vi "TCC_31_05_16_LIBRA.vi"() -> ()   [LabVIEW 2010]
doc: "Use this template to build a standard state machine design pattern. Each state executes code and determines which state to transition to. Contrast this design pattern with the User Interface Event Handler pattern, in which code executes in response to user actions. Contrast this design pattern also with the Queued Message Handler pattern, in which each message handling code can queue zero or more new messages."
uses:
  TCC_01_02_15.ctl
  <vilib>/Instr/_visa.llb/VISA Configure Serial Port (Instr).vi
  <vilib>/Utility/file.llb/Write To Spreadsheet File (DBL).vi
  <vilib>/Analysis/NI_AALBase.lvlib
panel:
  out "Quantidade de Passos N-1":sgl
  in  "port":u16=20551
  out "Resulting string (W)":string
  in  "COM PIC":refnum<visa-resource-name>
  in  "Quit":bool
  in  "Inicia Controle":bool
  out "Diferença em %":dbl
  in  "Potência max Laser":dbl
  out "Meter Serial Number 8":string
  in  "Location of FieldMax2Lib.dll in 8":path=path "C:/Windows/System32/FieldMax2Lib.dll"
  out "Meter Serial Number 7":string
  in  "Location of FieldMax2Lib.dll in 7":path=path "C:/Windows/System32/FieldMax2Lib.dll"
  out "Meter Serial Number 6":string
  out "Mínima Pot":dbl=0.009
  out "Meter Serial Number 5":string
  in  "Location of FieldMax2Lib.dll in 5":path=path "C:/Windows/System32/FieldMax2Lib.dll"
  out "Meter Serial Number 4":string
  in  "Location of FieldMax2Lib.dll in 4":path=path "C:/Windows/System32/FieldMax2Lib.dll"
  out "Meter Serial Number 3":string
  out "Motor Sensor":bool
  out "Motor Disco":bool
  out "Shutter ON (Verde)/ OFF (Vermelho)":bool
  out "Measurement\n (W)":dbl format="%0.8f"
  out "Desv.Padrão":dbl format="%.8f"
  out "Quantidade de Passos":sgl
  in  "Medida (W)":dbl=0.027000000700354576 min=0.027000000700354576 max=0.27000001072883606 step=0.0005000000237487257 format="%0.8f"
  in  "Setpoint (W)":dbl=0.027000000700354576 min=0.027000000700354576 max=0.27000001072883606 step=0.0005000000237487257
  out "i":i32
  out "Medida N-1 (W)":dbl=0.027000000700354576 min=0.027000000700354576 max=0.27000001072883606 step=0.0005000000237487257 format="%0.8f"
  out "DeltaP":dbl
  out "Coeficiente novo":dbl
  out "Inicia\nAutomático":bool
  in  "Mensagem de erro renviada":string
  out "Máxima Pot":dbl=0.145
  in  "service name":string="localhost"
  out "FS/AS?":string
  out "connection P3D ID out":refnum<k5>
  out "Erro TCP 3DP":errorcluster
  in  "Location of FieldMax2Lib.dll in 6":path=path "C:/Windows/System32/FieldMax2Lib.dll"
  out "Erro comando PIC":errorcluster
  in  "Location of FieldMax2Lib.dll in 3":path=path "C:/Windows/System32/FieldMax2Lib.dll"
  out "Comandos para o PIC":string
  out "return count":u32
  out "data out":string
  out "bytes written":i32
  out "Loop  2":i32
  out "initialized array  2":sgl[](array[numeric]) format="%#_8g"
  out "Loop":i32
  out "initialized array":sgl[](array[numeric]) format="%#_8g"
  out "N_passos string":string
  # "- Entradas do programa:"
  # "-Indicadores:"
  # "- Informações do medidor:"
  # "- Variáveis auxiliares:"
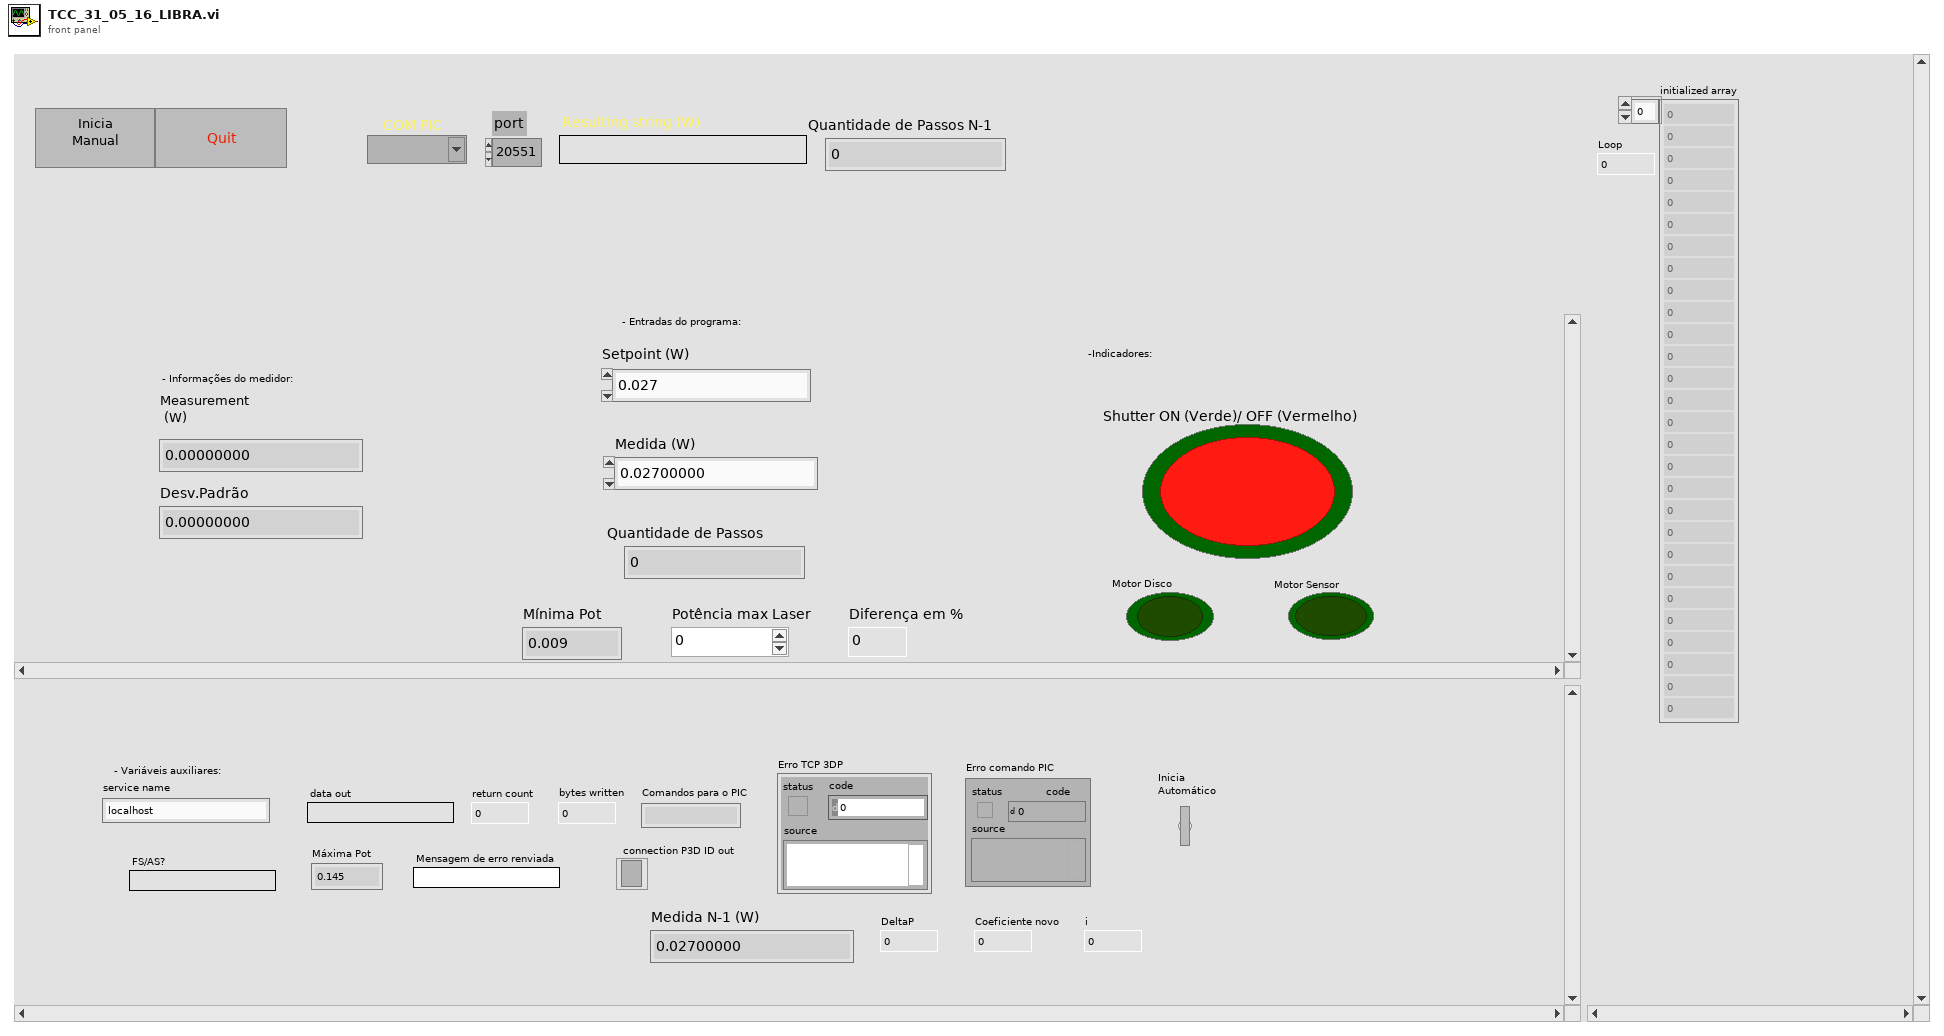
[diagram p1: front panel]
types:
  T1 = typedef "TCC_01_02_15.ctl" = enum16{"Receber Potencia", "Eventos", "Limites_P3D", "Limites_Manual", "Apenas Shutter", "Ajuste Manual", "Ajuste de Potência", "Stop"}
  T2 = enum8{"Enabled", "Disabled", "Disabled and Grayed Out"}
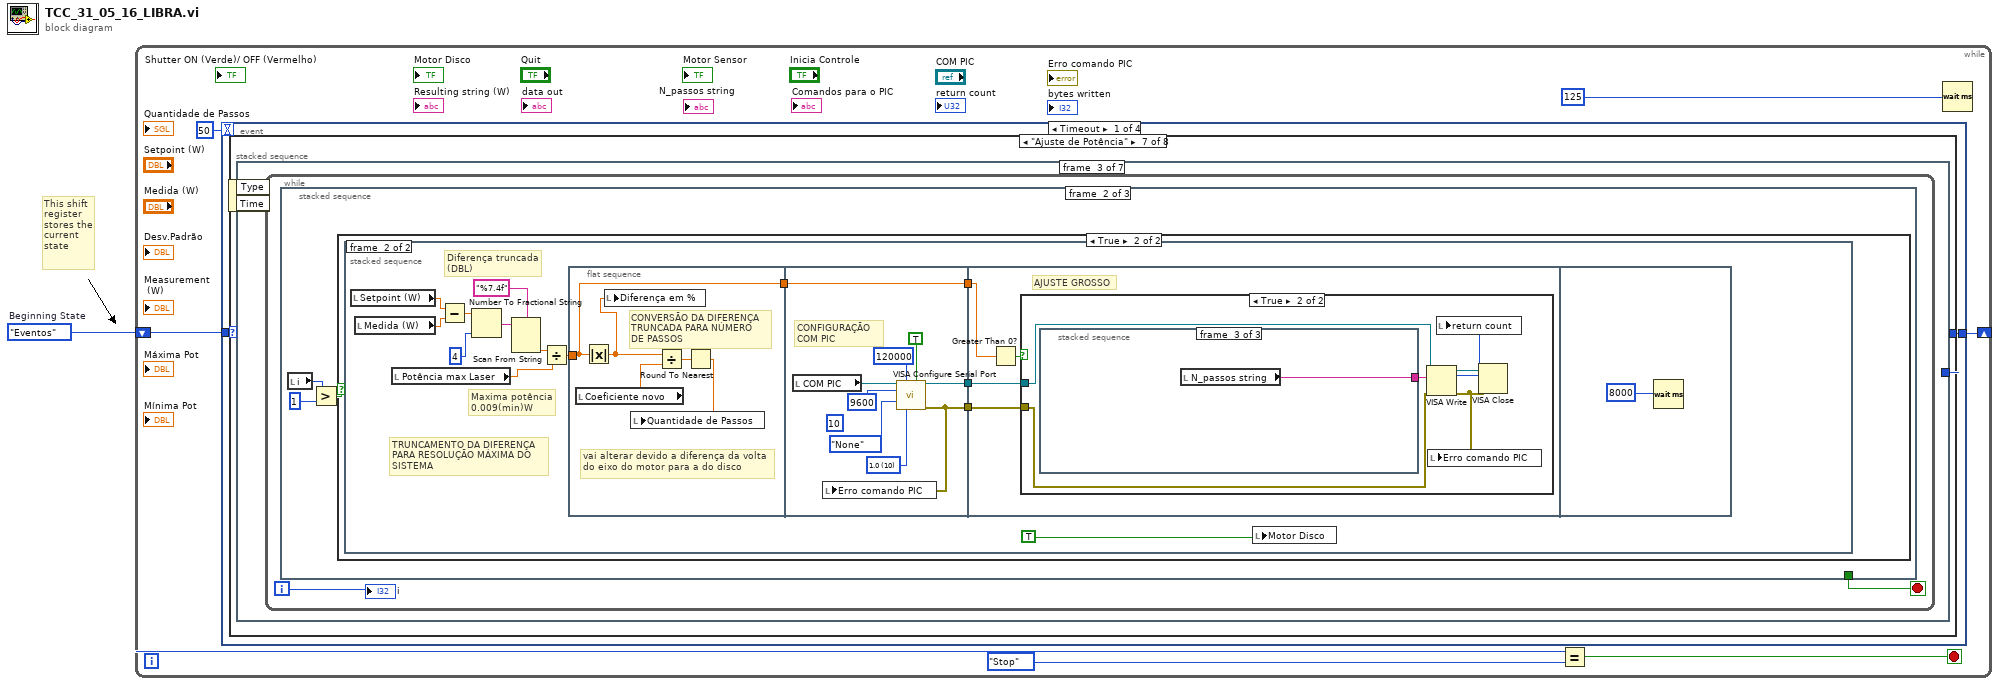
[diagram p0: block diagram]
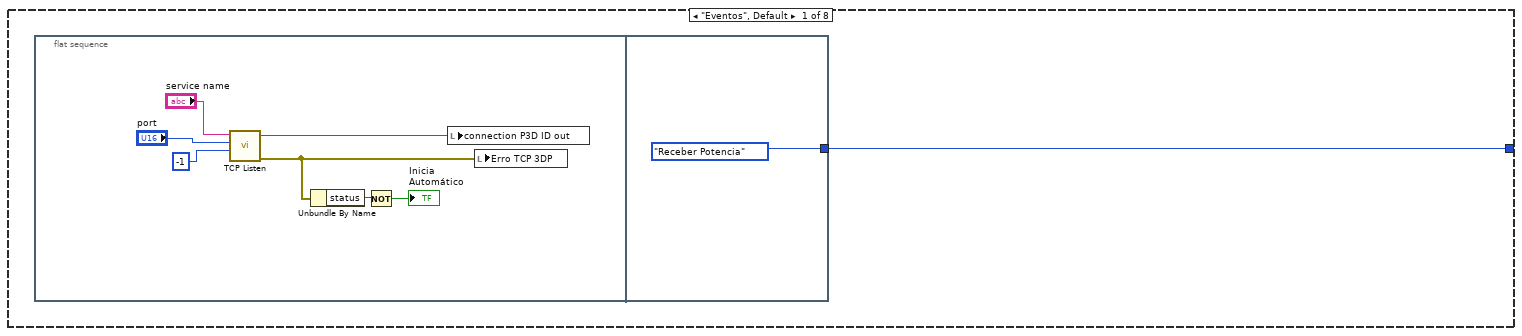
[diagram p2: hidden frame]
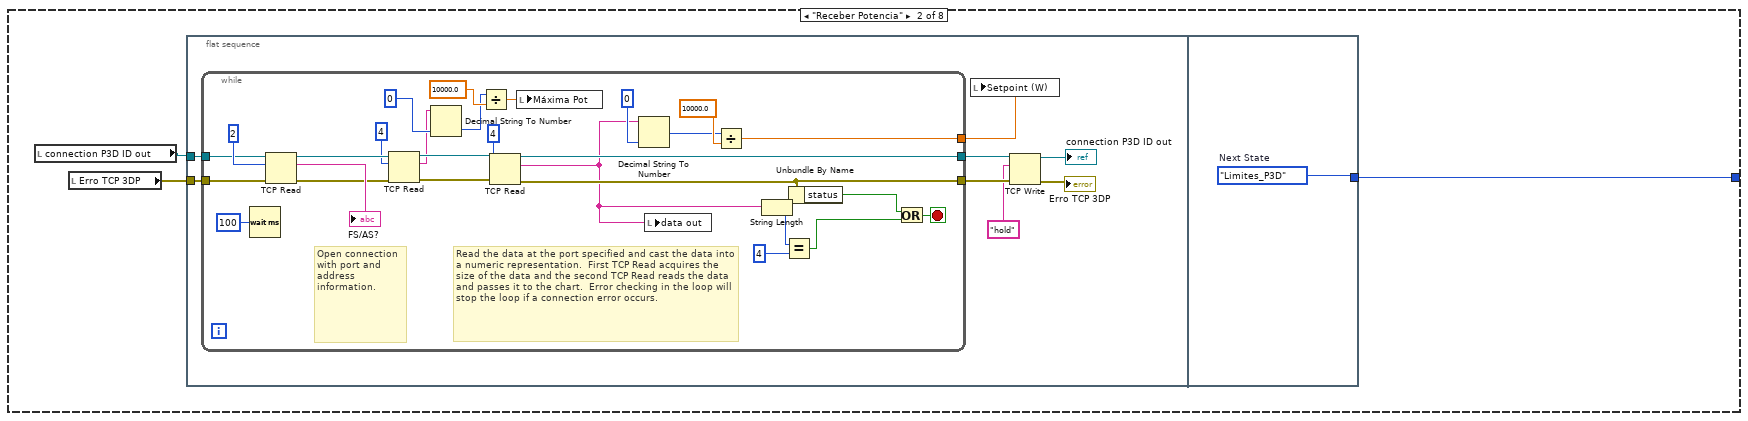
[diagram p3: hidden frame]
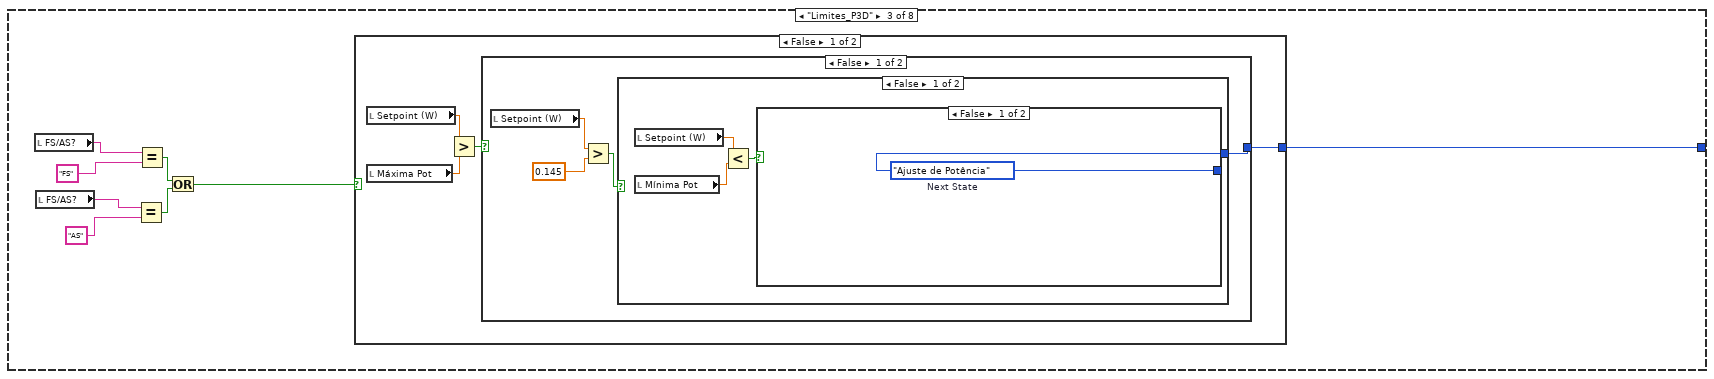
[diagram p4: hidden frame]
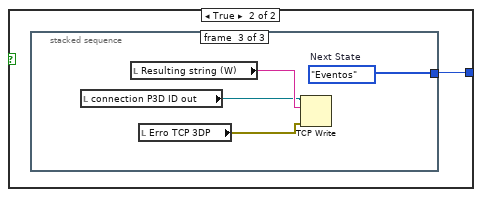
[diagram p5: hidden frame]
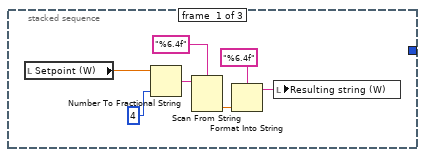
[diagram p6: hidden frame]
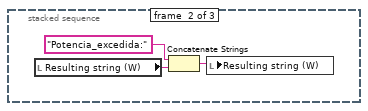
[diagram p7: hidden frame]
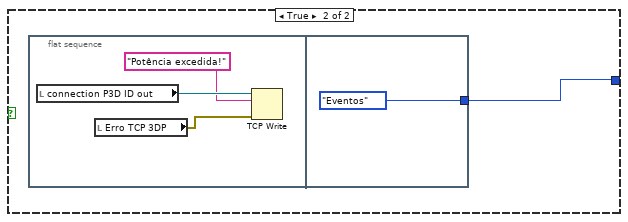
[diagram p8: hidden frame]
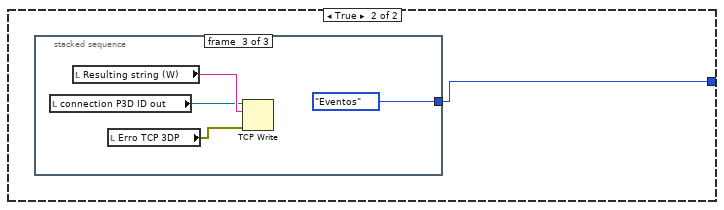
[diagram p9: hidden frame]
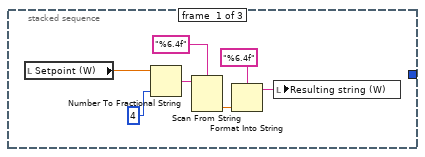
[diagram p10: hidden frame]
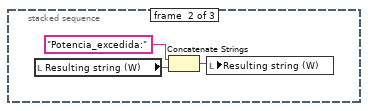
[diagram p11: hidden frame]
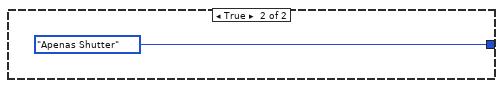
[diagram p12: hidden frame]
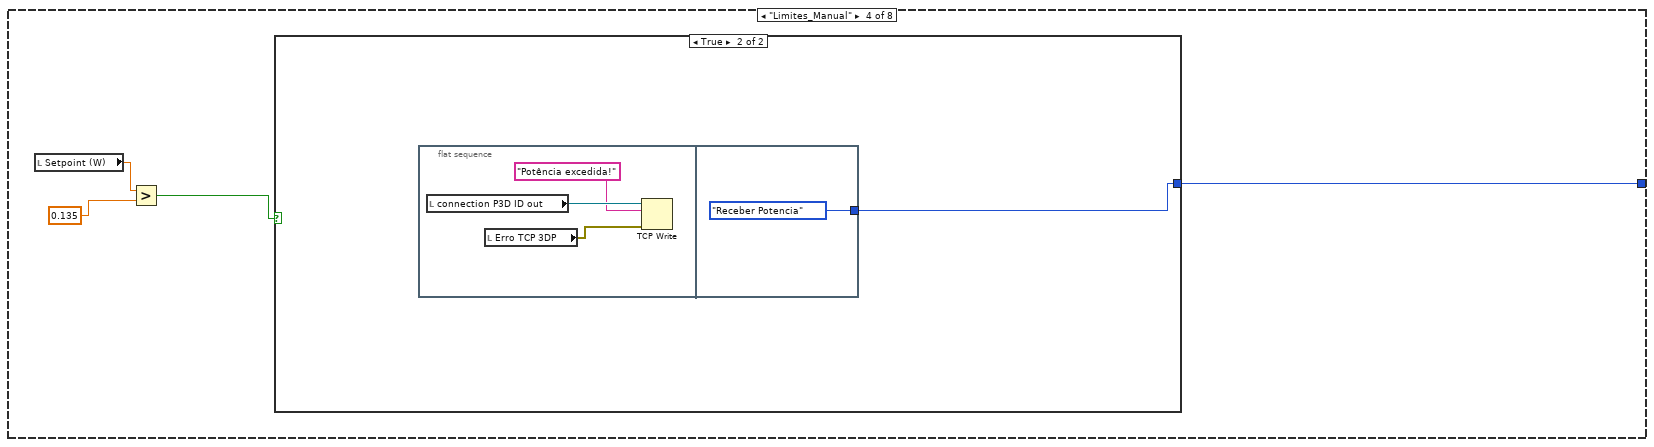
[diagram p13: hidden frame]
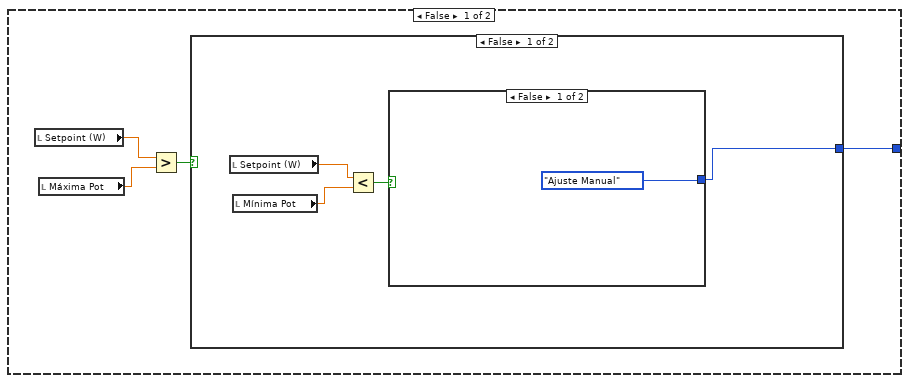
[diagram p14: hidden frame]
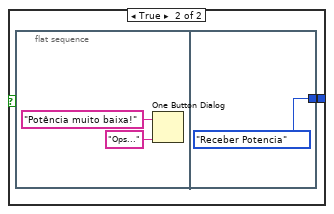
[diagram p15: hidden frame]
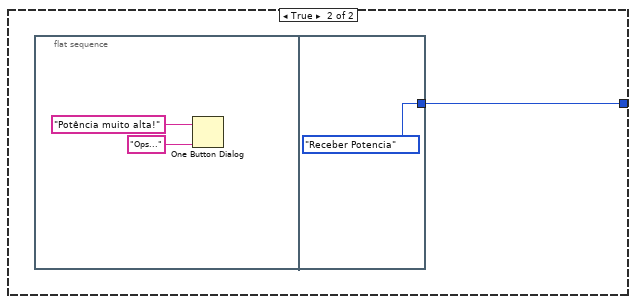
[diagram p16: hidden frame]
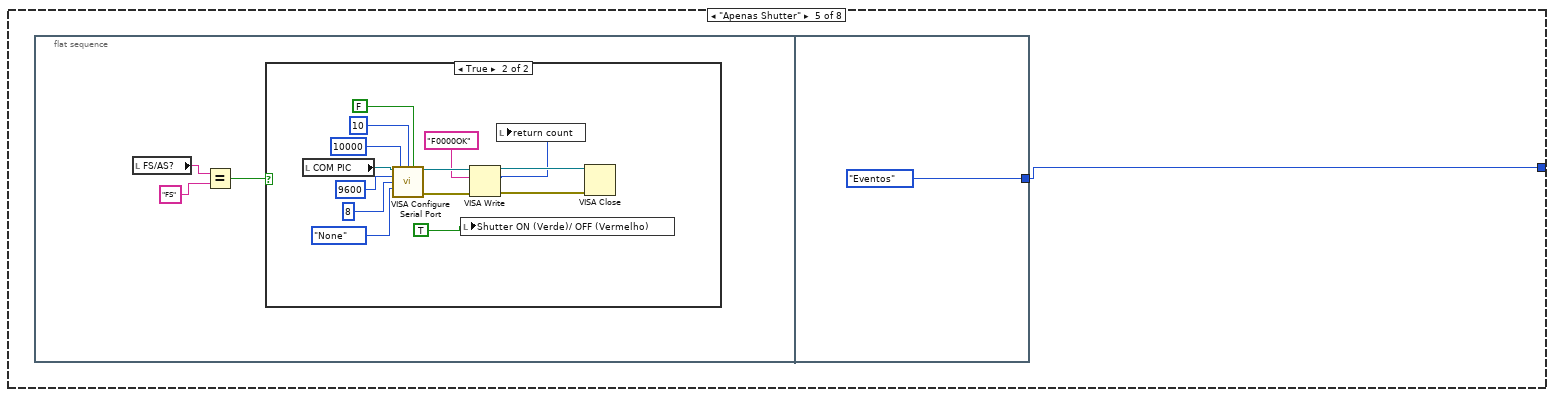
[diagram p17: hidden frame]
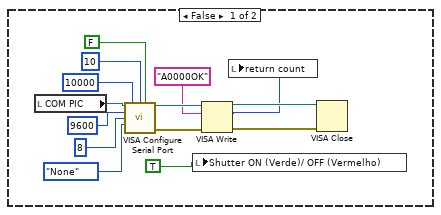
[diagram p18: hidden frame]
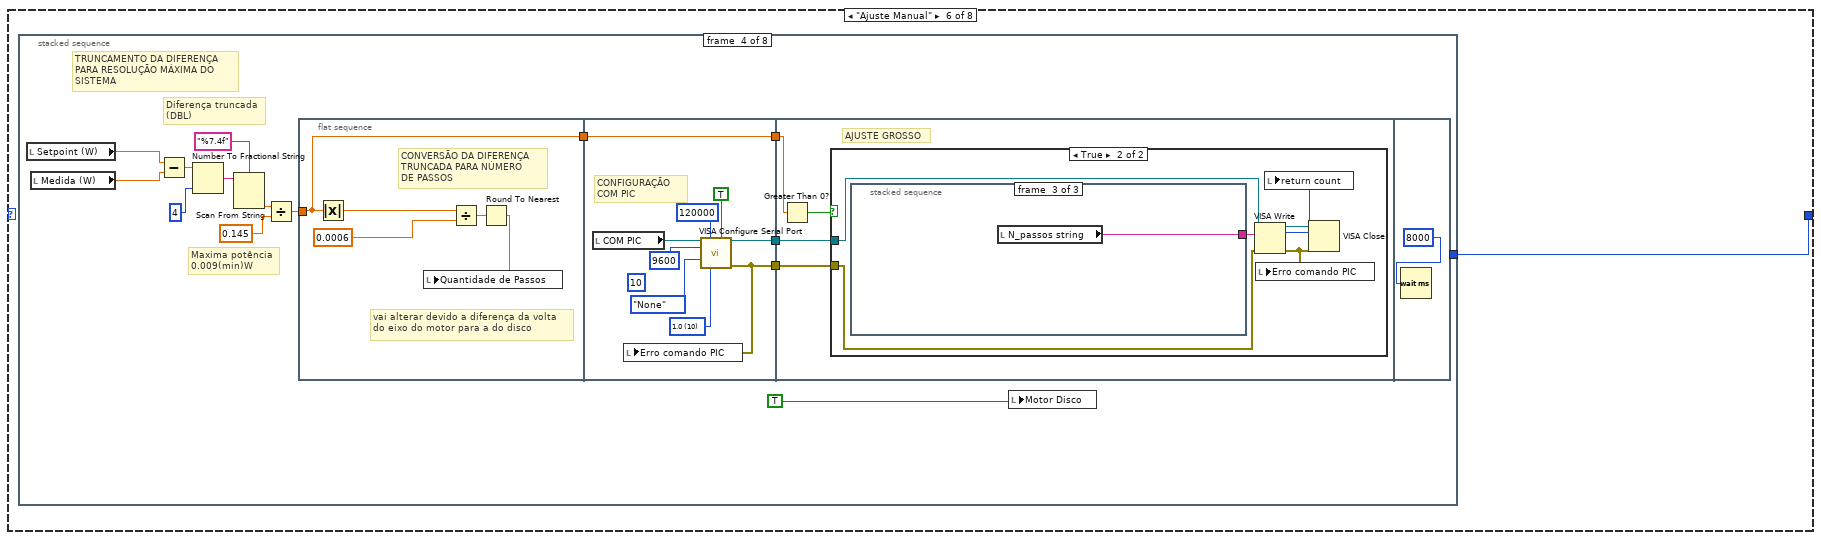
[diagram p19: hidden frame]
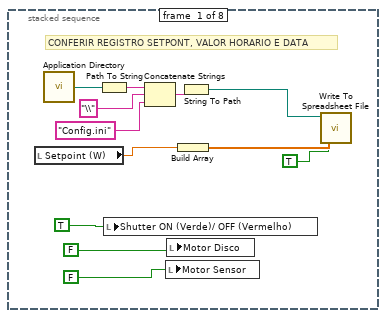
[diagram p20: hidden frame]
diagram:
  w1 = TCC_01_02_15."Eventos"  # Beginning State
  # "This shift\nregister\nstores the\ncurrent\nstate"
  n1 = while {
    shift-right: [w4] -> _
    shift-left: w1 -> [w5]
    stop <- w7 stop-if-true
    n2 = event shown="[0] Timeout" {
      selector: _ -> [_ _ _ _]
      dyn-events: _ -> [_ _ _ _]
      timeout: 50 -> [_ _ _ _]
      tunnel: w5 -> [w9 _ _ _]
      tunnel: [w8 w1061 TCC_01_02_15."Stop" ("States") w1068] -> w4
      event Timeout {
        n3 = event-data() -> ()  [unwired: 1 in, 2 out]
        n4 = case shown="\"Ajuste de Potência\"" w9 {
          tunnel: [w10 w21 w66 w119 w142 w175 w539 TCC_01_02_15."Eventos" ("Next State")] -> w8
          frame "Eventos", Default {
            n5 = flat-sequence {
              tunnel: [TCC_01_02_15."Receber Potencia" ("States")] -> w10
              frame #0 {
                n6 = call <vilib>:"TCP Listen.vi"("timeout ms (wait forever: -1)"=-1, "port"="port", "service name"="service name") -> ("error out"=w12:errorcluster, "connection ID"=w11:refnum<k5>)  [unwired: 5 in, 2 out]
                n7 = Unbundle By Name(w12) -> ("status"=w14:bool)
                n8 = Not(x=w14) -> (.not. x?=→"Inicia\nAutomático":bool)
                n9 = local write "connection P3D ID out"(w11) -> ()
                n10 = local write "Erro TCP 3DP"(w12) -> ()
              }
              frame #1 {
              }
            }
          }
          frame "Receber Potencia" {
            n11 = local read "connection P3D ID out"() -> (w19:refnum<k5>)
            n12 = local read "Erro TCP 3DP"() -> (w20:errorcluster)
            n13 = flat-sequence {
              tunnel: w19 -> [w23]
              tunnel: w20 -> [w22]
              tunnel: [w58] -> w21
              frame #0 {
                n14 = while {
                  tunnel: [w46] -> w28
                  tunnel: [w47] -> w29
                  tunnel: w23 -> [w53]
                  tunnel: w22 -> [w52]
                  tunnel: [w51] -> w26
                  stop <- w40 stop-if-true
                  # "Read the data at the port specified and cast the data into a numeric representation.  First TCP Read acquires the size of the data and the second TCP Read reads the data and passes it to the chart.  Error checking in the loop will stop the loop if a connection error occurs."
                  # "Open connection\nwith port and \naddress information."
                  n15 = Wait (ms)(milliseconds to wait=u32 100) -> ()  [unwired: 1 out]
                  n16 = TCP Read(connection ID=w53, bytes to read=2, error in (no error)=w52) -> (connection ID out=w38:refnum<k5>, data out=→"FS/AS?":string, error out=w39:errorcluster)  [unwired: 2 in]
                  n17 = TCP Read(connection ID=w38, bytes to read=4, error in (no error)=w39) -> (connection ID out=w37:refnum<k5>, data out=w34:string, error out=w36:errorcluster)  [unwired: 2 in]
                  n18 = Decimal String To Number(string=w34, default (0L)=0 ("default (0 I32)")) -> (number=w32:i32)  [unwired: 1 in, 1 out]
                  n19 = Divide(x=w32, y=10000.0) -> (x/y=w31:dbl)
                  n20 = TCP Read(connection ID=w37, bytes to read=u32 4, error in (no error)=w36) -> (connection ID out=w47:refnum<k5>, data out=w42:string, error out=w46:errorcluster)  [unwired: 2 in]
                  n21 = local write "Máxima Pot"(w31) -> ()
                  n22 = Decimal String To Number(string=w42, default (0L)=u32 0 ("default (0 I32)")) -> (number=w44:u32)  [unwired: 1 in, 1 out]
                  n23 = local write "data out"(w42) -> ()
                  n24 = Divide(x=w44, y=10000.0) -> (x/y=w51:dbl)
                  n25 = String Length(string=w42) -> (length=w43:i32)
                  n26 = Equal?(x=w43, y=4) -> (x = y?=w49:bool)
                  n27 = Unbundle By Name(w46) -> ("status"=w57:bool)
                  n28 = Or(x=w57, y=w49) -> (x .or. y?=w40:bool)
                }
                n29 = local write "Setpoint (W)"(w26) -> ()
                n30 = TCP Write(connection ID=w29, data in="hold", error in (no error)=w28) -> (connection ID out=→"connection P3D ID out":refnum<k5>, error out=→"Erro TCP 3DP":errorcluster)  [unwired: 1 in, 1 out]
              }
              frame #1 {
                w58 = TCC_01_02_15."Limites_P3D"  # Next State
              }
            }
          }
          frame "Limites_P3D" {
            n31 = local read "FS/AS?"() -> (w59:string)
            n32 = local read "FS/AS?"() -> (w60:string)
            n33 = Equal?(x=w60, y="AS") -> (x = y?=w62:bool)
            n34 = Equal?(x=w59, y="FS") -> (x = y?=w64:bool)
            n35 = Or(x=w64, y=w62) -> (x .or. y?=w61:bool)
            n36 = case shown="False" w61 {
              tunnel: [w67 TCC_01_02_15."Apenas Shutter" ("States")] -> w66
              frame False {
                n37 = local read "Setpoint (W)"() -> (w69:dbl)
                n38 = local read "Máxima Pot"() -> (w70:dbl)
                n39 = Greater?(x=w69, y=w70) -> (0:w68:bool)
                n40 = case shown="False" w68 {
                  tunnel: [w74 w100] -> w67
                  frame False {
                    n41 = local read "Setpoint (W)"() -> (w72:dbl)
                    n42 = Greater?(x=w72, y=0.145) -> (0:w71:bool)
                    n43 = case shown="False" w71 {
                      tunnel: [w75 w95] -> w74
                      frame False {
                        n44 = local read "Setpoint (W)"() -> (w78:dbl)
                        n45 = local read "Mínima Pot"() -> (w77:dbl)
                        n46 = Less?(x=w78, y=w77) -> (x < y?=w76:bool)
                        n47 = case shown="False" w76 {
                          tunnel: [w79 w80] -> w75
                          frame False {
                            w79 = TCC_01_02_15."Ajuste de Potência"  # Next State
                          }
                          frame True {
                            n48 = stacked-sequence {
                              tunnel: [_ _ w93] -> w80
                              frame #0 {
                                n49 = local read "Setpoint (W)"() -> (w84:dbl)
                                n50 = Number To Fractional String(number=w84, precision (6)=i16 4) -> (F-format string=w85:string)  [unwired: 2 in]
                                n51 = Scan From String(format string="%6.4f", input string=w85) -> (output 1=w81:dbl)  [unwired: 3 in, 3 out]
                                n52 = Format Into String(format string="%6.4f", w81) -> (resulting string=w82:string)  [unwired: 2 in, 1 out]
                                n53 = local write "Resulting string (W)"(w82) -> ()
                              }
                              frame #1 {
                                n54 = local read "Resulting string (W)"() -> (w90:string)
                                n55 = Concatenate Strings("Potencia_excedida:", w90) -> (w88:string)
                                n56 = local write "Resulting string (W)"(w88) -> ()
                              }
                              frame #2 {
                                w93 = TCC_01_02_15."Eventos"  # Next State
                                n57 = local read "connection P3D ID out"() -> (w92:refnum<k5>)
                                n58 = local read "Resulting string (W)"() -> (w94:string)
                                n59 = local read "Erro TCP 3DP"() -> (w91:errorcluster)
                                n60 = TCP Write(connection ID=w92, data in=w94, error in (no error)=w91) -> ()  [unwired: 1 in, 3 out]
                              }
                            }
                          }
                        }
                      }
                      frame True {
                        n61 = flat-sequence {
                          tunnel: [TCC_01_02_15."Eventos" ("States")] -> w95
                          frame #0 {
                            n62 = local read "connection P3D ID out"() -> (w97:refnum<k5>)
                            n63 = local read "Erro TCP 3DP"() -> (w98:errorcluster)
                            n64 = TCP Write(connection ID=w97, data in="Potência excedida!", error in (no error)=w98) -> ()  [unwired: 1 in, 3 out]
                          }
                          frame #1 {
                          }
                        }
                      }
                    }
                  }
                  frame True {
                    n65 = stacked-sequence {
                      tunnel: [_ _ TCC_01_02_15."Eventos" ("States")] -> w100
                      frame #0 {
                        n66 = local read "Setpoint (W)"() -> (w104:dbl)
                        n67 = Number To Fractional String(number=w104, precision (6)=i16 4) -> (F-format string=w105:string)  [unwired: 2 in]
                        n68 = Scan From String(format string="%6.4f", input string=w105) -> (output 1=w101:dbl)  [unwired: 3 in, 3 out]
                        n69 = Format Into String(format string="%6.4f", w101) -> (resulting string=w102:string)  [unwired: 2 in, 1 out]
                        n70 = local write "Resulting string (W)"(w102) -> ()
                      }
                      frame #1 {
                        n71 = local read "Resulting string (W)"() -> (w110:string)
                        n72 = Concatenate Strings("Potencia_excedida:", w110) -> (w108:string)
                        n73 = local write "Resulting string (W)"(w108) -> ()
                      }
                      frame #2 {
                        n74 = local read "connection P3D ID out"() -> (w111:refnum<k5>)
                        n75 = local read "Resulting string (W)"() -> (w114:string)
                        n76 = local read "Erro TCP 3DP"() -> (w112:errorcluster)
                        n77 = TCP Write(connection ID=w111, data in=w114, error in (no error)=w112) -> ()  [unwired: 1 in, 3 out]
                      }
                    }
                  }
                }
              }
              frame True {
              }
            }
          }
          frame "Limites_Manual" {
            n78 = local read "Setpoint (W)"() -> (w118:dbl)
            n79 = Greater?(x=w118, y=0.135) -> (0:w116:bool)
            n80 = case shown="True" w116 {
              tunnel: [w120 w137] -> w119
              frame False {
                n81 = local read "Setpoint (W)"() -> (w123:dbl)
                n82 = local read "Máxima Pot"() -> (w122:dbl)
                n83 = Greater?(x=w123, y=w122) -> (0:w121:bool)
                n84 = case shown="False" w121 {
                  tunnel: [w124 w133] -> w120
                  frame False {
                    n85 = local read "Setpoint (W)"() -> (w126:dbl)
                    n86 = local read "Mínima Pot"() -> (w127:dbl)
                    n87 = Less?(x=w126, y=w127) -> (x < y?=w125:bool)
                    n88 = case shown="False" w125 {
                      tunnel: [TCC_01_02_15."Ajuste Manual" ("States") w129] -> w124
                      frame False {
                      }
                      frame True {
                        n89 = flat-sequence {
                          tunnel: [TCC_01_02_15."Receber Potencia" ("States")] -> w129
                          frame #0 {
                            n90 = One Button Dialog(message="Potência muito baixa!", button name ("OK")="Ops...") -> ()  [unwired: 1 out]
                          }
                          frame #1 {
                          }
                        }
                      }
                    }
                  }
                  frame True {
                    n91 = flat-sequence {
                      tunnel: [TCC_01_02_15."Receber Potencia" ("States")] -> w133
                      frame #0 {
                        n92 = One Button Dialog(message="Potência muito alta!", button name ("OK")="Ops...") -> ()  [unwired: 1 out]
                      }
                      frame #1 {
                      }
                    }
                  }
                }
              }
              frame True {
                n93 = flat-sequence {
                  tunnel: [TCC_01_02_15."Receber Potencia" ("States")] -> w137
                  frame #0 {
                    n94 = local read "connection P3D ID out"() -> (w139:refnum<k5>)
                    n95 = local read "Erro TCP 3DP"() -> (w140:errorcluster)
                    n96 = TCP Write(connection ID=w139, data in="Potência excedida!", error in (no error)=w140) -> ()  [unwired: 1 in, 3 out]
                  }
                  frame #1 {
                  }
                }
              }
            }
          }
          frame "Apenas Shutter" {
            n97 = flat-sequence {
              tunnel: [TCC_01_02_15."Eventos" ("States")] -> w142
              frame #0 {
                n98 = local read "FS/AS?"() -> (w145:string)
                n99 = Equal?(x=w145, y="FS") -> (x = y?=w143:bool)
                n100 = case shown="True" w143 {
                  frame False {
                    n101 = local read "COM PIC"() -> (w152:refnum<visa-resource-name>)
                    n102 = call-poly "VISA Configure Serial Port"("VISA resource name"=w152, "timeout (10sec)"=u32 10000, "termination char\n(0xA = '\\n' = LF)"=u8 10 ("termination char\n(0xA = '\\n' = LF)"), "Enable Termination\nChar (T)"=FALSE ("Enable Termination\nChar (T)"), "baud rate (9600)"=u32 9600, "data bits (8)"=u16 8, "parity (0:none)"=enum16{"None", "Odd", "Even", "Mark", "Space"}."None") -> ("VISA resource name out"=w151:refnum<visa-resource-name>, "error out"=w150:errorcluster)  [unwired: 7 in]
                    n103 = local write "Shutter ON (Verde)/ OFF (Vermelho)"(TRUE ("Inicia Controle")) -> ()
                    n104 = VISA Write(VISA resource name=w151, write buffer="A0000OK", error in (no error)=w150) -> (VISA resource name out=w147:refnum<visa-resource-name>, return count=w146:u32, error out=w148:errorcluster)
                    n105 = local write "return count"(w146) -> ()
                    n106 = VISA Close(VISA resource name=w147, error in (no error)=w148) -> ()  [unwired: 1 out]
                  }
                  frame True {
                    n107 = local read "COM PIC"() -> (w166:refnum<visa-resource-name>)
                    n108 = call-poly "VISA Configure Serial Port"("VISA resource name"=w166, "timeout (10sec)"=u32 10000, "termination char\n(0xA = '\\n' = LF)"=u8 10 ("termination char\n(0xA = '\\n' = LF)"), "Enable Termination\nChar (T)"=FALSE ("Enable Termination\nChar (T)"), "baud rate (9600)"=u32 9600, "data bits (8)"=u16 8, "parity (0:none)"=enum16{"None", "Odd", "Even", "Mark", "Space"}."None") -> ("VISA resource name out"=w165:refnum<visa-resource-name>, "error out"=w164:errorcluster)  [unwired: 7 in]
                    n109 = local write "Shutter ON (Verde)/ OFF (Vermelho)"(TRUE ("Inicia Controle")) -> ()
                    n110 = VISA Write(VISA resource name=w165, write buffer="F0000OK", error in (no error)=w164) -> (VISA resource name out=w161:refnum<visa-resource-name>, return count=w160:u32, error out=w162:errorcluster)
                    n111 = local write "return count"(w160) -> ()
                    n112 = VISA Close(VISA resource name=w161, error in (no error)=w162) -> ()  [unwired: 1 out]
                  }
                }
              }
              frame #1 {
              }
            }
          }
          frame "Ajuste Manual" {
            n113 = stacked-sequence {
              tunnel: [_ _ _ _ _ _ _ TCC_01_02_15."Eventos" ("States")] -> w175
              frame #0 {
                # "CONFERIR REGISTRO SETPONT, VALOR HORARIO E DATA"
                n114 = local read "Setpoint (W)"() -> (w180:dbl)
                n115 = call <vilib>:"Application Directory.vi"() -> ("Application Directory"=w187:path)
                n116 = Path To String(path=w187) -> (string=w185:string)
                n117 = local write "Shutter ON (Verde)/ OFF (Vermelho)"(TRUE) -> ()
                n118 = Concatenate Strings(w185, "\\" ("string"), "Config.ini" ("replace string (\"\")")) -> (w186:string)
                n119 = local write "Motor Sensor"(FALSE) -> ()
                n120 = local write "Motor Disco"(FALSE) -> ()
                n121 = Build Array(w180) -> (w183:dbl[])
                n122 = String To Path(string=w186) -> (path=w184:path)
                n123 = call-poly <vilib>:"Write To Spreadsheet File.vi"("append to file? (new file:F)"=TRUE, "1D data"=w183, "file path (dialog if empty)"=w184) -> ()  [unwired: 5 in, 1 out]
              }
              frame #1 {
                n124 = flat-sequence {
                  tunnel: [w203] -> w191
                  tunnel: [w201] -> w189
                  tunnel: w191 -> [w214]
                  tunnel: [w214] -> w190
                  tunnel: w189 -> [w213]
                  tunnel: [w213] -> w188
                  tunnel: w190 -> [w218]
                  tunnel: w188 -> [w219]
                  tunnel: [w216] -> w199
                  tunnel: [w215] -> w198
                  tunnel: w199 -> [w229]
                  tunnel: w198 -> [w228]
                  tunnel: [w226] -> w197
                  tunnel: [w225] -> w196
                  tunnel: w197 -> [w237]
                  tunnel: w196 -> [w236]
                  tunnel: [w235] -> w194
                  tunnel: [w234] -> w192
                  tunnel: [w242] -> w195
                  tunnel: w194 -> [w242]
                  tunnel: [w241] -> w193
                  tunnel: w192 -> [w241]
                  tunnel: w195 -> [w245]
                  tunnel: w193 -> [w244]
                  frame #0 {
                    w202 = u16 10 items=["1.0"=10, "1.5"=15, "2.0"=20] ("stop bits (10: 1 bit)")
                    (unwired) u32 120000 ("timeout (10sec)")
                    (unwired) u16 10 ("data bits (8)")
                    # "CONFIGURAÇÃO COMUNICAÇÃO PIC"
                    n125 = local read "COM PIC"() -> (w211:refnum<visa-resource-name>)
                    n126 = local write "Shutter ON (Verde)/ OFF (Vermelho)"(FALSE ("Inicia Controle")) -> ()
                    n127 = local write "Motor Disco"(FALSE) -> ()
                    n128 = local write "Motor Sensor"(FALSE) -> ()
                    n129 = call-poly "VISA Configure Serial Port"("VISA resource name"=w211, "termination char\n(0xA = '\\n' = LF)"=u8 13 ("termination char\n(0xA = '\\n' = LF)"), "Enable Termination\nChar (T)"=TRUE, "baud rate (9600)"=u32 9600, "parity (0:none)"=enum16{"None", "Odd", "Even", "Mark", "Space"}."None", "stop bits (10: 1 bit)"=w202) -> ("VISA resource name out"=w203:refnum<visa-resource-name>, "error out"=w201:errorcluster)  [unwired: 8 in]
                    n130 = local write "Erro comando PIC"(w201) -> ()
                  }
                  frame #1 {
                    n131 = Wait (ms)(milliseconds to wait=500) -> ()  [unwired: 1 out]
                  }
                  frame #2 {
                    # "FECHAMENTO OBTURADOR"
                    n132 = local write "Shutter ON (Verde)/ OFF (Vermelho)"(TRUE) -> ()
                    n133 = VISA Write(VISA resource name=w218, write buffer="F0000OK", error in (no error)=w219) -> (VISA resource name out=w216:refnum<visa-resource-name>, return count=w223:u32, error out=w215:errorcluster)
                    n134 = local write "return count"(w223) -> ()
                    n135 = local write "Motor Sensor"(FALSE) -> ()
                    n136 = local write "Motor Disco"(FALSE) -> ()
                    n137 = local write "Erro comando PIC"(w215) -> ()
                    n138 = Wait (ms)(milliseconds to wait=u32 1000) -> ()  [unwired: 1 out]
                  }
                  frame #3 {
                    # "POSICIONAMENTO SENSOR"
                    n139 = local write "Shutter ON (Verde)/ OFF (Vermelho)"(TRUE) -> ()
                    n140 = VISA Write(VISA resource name=w229, write buffer="P0000OK", error in (no error)=w228) -> (VISA resource name out=w226:refnum<visa-resource-name>, return count=w233:u32, error out=w225:errorcluster)
                    n141 = local write "return count"(w233) -> ()
                    n142 = local write "Motor Sensor"(TRUE) -> ()
                    n143 = local write "Erro comando PIC"(w225) -> ()
                    n144 = Wait (ms)(milliseconds to wait=u32 2000) -> ()  [unwired: 1 out]
                  }
                  frame #4 {
                    # "ABERTURA DO OBTURADOR E HOLD-OFF\n ESTABILIAZAÇÃO SENSOR"
                    n145 = local write "Shutter ON (Verde)/ OFF (Vermelho)"(FALSE) -> ()
                    n146 = VISA Write(VISA resource name=w237, write buffer="A0000OK", error in (no error)=w236) -> (VISA resource name out=w235:refnum<visa-resource-name>, return count=w240:u32, error out=w234:errorcluster)
                    n147 = local write "return count"(w240) -> ()
                    n148 = local write "Erro comando PIC"(w234) -> ()
                  }
                  frame #5 {
                    # "Atraso após\nestabilidade\ntérmica"
                    n149 = Wait (ms)(milliseconds to wait=u32 10000) -> ()  [unwired: 1 out]
                  }
                  frame #6 {
                    n150 = VISA Close(VISA resource name=w245, error in (no error)=w244) -> ()  [unwired: 1 out]
                  }
                }
                n151 = property on="Setpoint (W)" class="DigNum (strict)"("DisabledEnum"=T2."Disabled and Grayed Out" ("Disabled")) -> ()  [unwired: 2 in, 2 out]
              }
              frame #2 {
                n152 = flat-sequence {
                  frame #0 {
                    n153 = disable-structure shown="Disabled" {
                      frame Disabled {
                        # "AMOSTRAGEM INICIAL (20 VALORES)"
                        n154 = call "Connect_To_Meter.vi"("Location of FieldMax2Lib.dll in"="Location of FieldMax2Lib.dll in 6") -> ("Meter Serial Number"=→"Meter Serial Number 6":string, "Meter ID out"=w248:i32, "Location of FieldMax2Lib.dll out"=w249:path)  [unwired: 6 in]
                        n155 = dll-call lib="C:/Windows/System32/FieldMax2Lib.dll" fn="fm2LibSync" label="Sync"(path in=w249, "h"=w248) -> (path out=w247:path, "h"=w246:i32)  [unwired: 3 in, 1 out]
                        n156 = Initialize Array(u8 0 ("element"), 64 ("dimension size")) -> (w255:u8[])
                        n157 = for {
                          N: 21 -> [_]
                          tunnel: w246 -> [w264]
                          tunnel: w255 -> [w270]
                          tunnel: i16 8 ("count") -> [w269]
                          tunnel: [w266] -> w251
                          tunnel: w247 -> [w271]
                          tunnel: [w265] -> w250
                          shift-right: [w261] -> w259
                          shift-left: sgl[] [] -> [w262]
                          i -> [w263]
                          n158 = dll-call lib="C:/Windows/System32/FieldMax2Lib.dll" fn="fm2LibGetData" label="Get Data"(path in=w271, "h"=w264, "returnBuffer"=w270, "count"=w269) -> (path out=w265:path, "h"=w266:i32, "returnBuffer"=w267:u8[], "count"=w268:i16)  [unwired: 3 in, 1 out]
                          n159 = Not Equal To 0?(x=w268) -> (x != 0?=w272:bool)
                          n160 = call "Utility - Bytes to Values.vi"("DataBuffer"=w267) -> ("Measurement Value"=w273:sgl)  [unwired: 9 in, 1 out]
                          n161 = Wait (ms)(milliseconds to wait=u32 1000) -> ()  [unwired: 1 out]
                          n162 = case shown="True" w272 {
                            tunnel: w273 -> [w276 w277]
                            tunnel: [w276 w277] -> _
                            tunnel: w262 -> [w275 w279]
                            tunnel: [w275 w278] -> w261
                            frame False {
                              (unwired) FALSE
                            }
                            frame True {
                              n163 = local write "Measurement\n (W)"(w277) -> ()
                              n164 = Build Array (concatenate)(w279, w277) -> (w278:sgl[])
                            }
                          }
                          "Loop  2" <- w263
                        }
                        "initialized array  2" <- w259
                        n165 = call "Disconnect_From_Meter.vi"("Location of FieldMax2Lib.dll in"=w250, "Meter ID in"=w251) -> ()  [unwired: 7 in, 2 out]
                      }
                      frame Enabled {
                        n166 = local write "Medida (W)"(0.105 ("Measurement")) -> ()
                      }
                    }
                  }
                  frame #1 {
                    # "CALCULO DO VALOR MEDIO DA BATERIA DE\nVALORES E SEU DESVIO PADRÃO (VALIDAÇÃO)"
                    n167 = disable-structure shown="Enabled" {
                      frame Disabled {
                        n168 = local read "initialized array  2"() -> (w281:sgl[])
                        n169 = call <vilib>:"Std Deviation and Variance.vi"("X"=w281, "Weighting (Sample)"=enum16{"Sample", "Population"}."Population") -> ("mean"=w284:dbl, "standard deviation"=w283:dbl)  [unwired: 1 out]
                        n170 = local write "Medida (W)"(w284) -> ()
                        n171 = local write "Desv.Padrão"(w283) -> ()
                      }
                      frame Enabled {
                      }
                    }
                  }
                }
              }
              frame #3 {
                # "TRUNCAMENTO DA DIFERENÇA \nPARA RESOLUÇÃO MÁXIMA DO\nSISTEMA"
                # "Maxima potência\n0.009(min)W"
                # "Diferença truncada\n(DBL)"
                n172 = local read "Setpoint (W)"() -> (w298:dbl)
                n173 = local read "Medida (W)"() -> (w297:dbl)
                n174 = Subtract(x=w298, y=w297) -> (x-y=w290:dbl)
                n175 = Number To Fractional String(number=w290, precision (6)=i16 4) -> (F-format string=w294:string)  [unwired: 2 in]
                n176 = Scan From String(format string="%7.4f", input string=w294) -> (output 1=w295:dbl)  [unwired: 3 in, 3 out]
                n177 = Divide(x=w295, y=0.145) -> (x/y=w289:dbl)
                n178 = flat-sequence {
                  tunnel: w289 -> [w299]
                  tunnel: [w299] -> w288
                  tunnel: w288 -> [w312]
                  tunnel: [w312] -> w287
                  tunnel: [w306] -> w286
                  tunnel: [w304] -> w285
                  tunnel: w287 -> [w315]
                  tunnel: w286 -> [w314]
                  tunnel: w285 -> [w313]
                  frame #0 {
                    # "CONVERSÃO DA DIFERENÇA\nTRUNCADA PARA NÚMERO\nDE PASSOS"
                    # "vai alterar devido a diferença da volta \ndo eixo do motor para a do disco"
                    n179 = Absolute Value(x=w299) -> (abs(x)=w300:dbl)
                    n180 = Divide(x=w300, y=0.0006) -> (x/y=w302:dbl)
                    n181 = Round To Nearest(number=w302) -> (nearest integer value=w303:dbl)
                    n182 = local write "Quantidade de Passos"(w303) -> ()
                  }
                  frame #1 {
                    w305 = u16 10 items=["1.0"=10, "1.5"=15, "2.0"=20] ("stop bits (10: 1 bit)")
                    (unwired) u16 10 ("data bits (8)")
                    # "CONFIGURAÇÃO \nCOM PIC"
                    n183 = local read "COM PIC"() -> (w307:refnum<visa-resource-name>)
                    n184 = call-poly "VISA Configure Serial Port"("VISA resource name"=w307, "timeout (10sec)"=u32 120000, "Enable Termination\nChar (T)"=TRUE, "baud rate (9600)"=u32 9600, "parity (0:none)"=enum16{"None", "Odd", "Even", "Mark", "Space"}."None", "stop bits (10: 1 bit)"=w305) -> ("VISA resource name out"=w306:refnum<visa-resource-name>, "error out"=w304:errorcluster)  [unwired: 8 in]
                    n185 = local write "Erro comando PIC"(w304) -> ()
                  }
                  frame #2 {
                    # "AJUSTE GROSSO"
                    n186 = Greater Than 0?(x=w315) -> (x > 0?=w316:bool)
                    n187 = case shown="True" w316 {
                      tunnel: w314 -> [w320 w344]
                      tunnel: w313 -> [w319 w345]
                      frame False {
                        n188 = stacked-sequence {
                          tunnel: [_ _ w341] -> w322
                          frame #0 {
                            n189 = local read "Quantidade de Passos"() -> (w323:sgl)
                            n190 = Format Into String(format string="%d", w323) -> (resulting string=w325:string)  [unwired: 2 in, 1 out]
                            n191 = String Length(string=w325) -> (length=w326:i32)
                            n192 = case shown="1, Default" w326 {
                              tunnel: w325 -> [w328 w331 w333 w336]
                              frame 1, Default {
                                n193 = Concatenate Strings("000" ("string"), w328) -> (w329:string)
                                n194 = local write "N_passos string"(w329) -> ()
                              }
                              frame 2 {
                                n195 = Concatenate Strings("00" ("string"), w331) -> (w330:string)
                                n196 = local write "N_passos string"(w330) -> ()
                              }
                              frame 3 {
                                n197 = Concatenate Strings("0" ("string"), w333) -> (w334:string)
                                n198 = local write "N_passos string"(w334) -> ()
                              }
                              frame 4 {
                                n199 = local write "N_passos string"(w336) -> ()
                              }
                            }
                          }
                          frame #1 {
                            # "adicionar letra"
                            n200 = local read "N_passos string"() -> (w338:string)
                            n201 = Concatenate Strings("D" ("string"), w338, "OK" ("string")) -> (w340:string)
                            n202 = local write "N_passos string"(w340) -> ()
                          }
                          frame #2 {
                            n203 = local read "N_passos string"() -> (w341:string)
                          }
                        }
                        n204 = VISA Write(VISA resource name=w320, write buffer=w322, error in (no error)=w319) -> (VISA resource name out=w318:refnum<visa-resource-name>, return count=w321:u32, error out=w317:errorcluster)
                        n205 = local write "Erro comando PIC"(w317) -> ()
                        n206 = local write "return count"(w321) -> ()
                        n207 = VISA Close(VISA resource name=w318, error in (no error)=w317) -> ()  [unwired: 1 out]
                      }
                      frame True {
                        n208 = stacked-sequence {
                          tunnel: [_ _ w366] -> w347
                          frame #0 {
                            n209 = local read "Quantidade de Passos"() -> (w348:sgl)
                            n210 = Format Into String(format string="%d", w348) -> (resulting string=w350:string)  [unwired: 2 in, 1 out]
                            n211 = String Length(string=w350) -> (length=w351:i32)
                            n212 = case shown="3" w351 {
                              tunnel: w350 -> [w352 w356 w358 w361]
                              frame 1, Default {
                                n213 = Concatenate Strings("000" ("string"), w352) -> (w354:string)
                                n214 = local write "N_passos string"(w354) -> ()
                              }
                              frame 2 {
                                n215 = Concatenate Strings("00" ("string"), w356) -> (w355:string)
                                n216 = local write "N_passos string"(w355) -> ()
                              }
                              frame 3 {
                                n217 = Concatenate Strings("0" ("string"), w358) -> (w359:string)
                                n218 = local write "N_passos string"(w359) -> ()
                              }
                              frame 4 {
                                n219 = local write "N_passos string"(w361) -> ()
                              }
                            }
                          }
                          frame #1 {
                            n220 = local read "N_passos string"() -> (w363:string)
                            n221 = Concatenate Strings("I" ("string"), w363, "OK" ("string")) -> (w365:string)
                            n222 = local write "N_passos string"(w365) -> ()
                          }
                          frame #2 {
                            n223 = local read "N_passos string"() -> (w366:string)
                          }
                        }
                        n224 = VISA Write(VISA resource name=w344, write buffer=w347, error in (no error)=w345) -> (VISA resource name out=w343:refnum<visa-resource-name>, return count=w346:u32, error out=w342:errorcluster)
                        n225 = local write "Erro comando PIC"(w342) -> ()
                        n226 = local write "return count"(w346) -> ()
                        n227 = VISA Close(VISA resource name=w343, error in (no error)=w342) -> ()  [unwired: 1 out]
                      }
                    }
                  }
                  frame #3 {
                    n228 = Wait (ms)(milliseconds to wait=8000) -> ()  [unwired: 1 out]
                  }
                }
                n229 = local write "Motor Disco"(TRUE) -> ()
              }
              frame #4 {
                n230 = flat-sequence {
                  tunnel: [w373] -> w369
                  tunnel: [w372] -> w368
                  tunnel: w369 -> [w380]
                  tunnel: w368 -> [w379]
                  frame #0 {
                    w371 = u16 10 items=["1.0"=10, "1.5"=15, "2.0"=20] ("stop bits (10: 1 bit)")
                    (unwired) u8 13 ("termination char\n(0xA = '\\n' = LF)")
                    (unwired) u16 10 ("data bits (8)")
                    # "CONFIGURAÇÃO COMUNICAÇÃO PIC"
                    n231 = local read "COM PIC"() -> (w378:refnum<visa-resource-name>)
                    n232 = Wait (ms)(milliseconds to wait=u32 3000) -> ()  [unwired: 1 out]
                    n233 = call-poly "VISA Configure Serial Port"("VISA resource name"=w378, "timeout (10sec)"=u32 120000, "Enable Termination\nChar (T)"=TRUE, "baud rate (9600)"=u32 9600, "parity (0:none)"=enum16{"None", "Odd", "Even", "Mark", "Space"}."None", "stop bits (10: 1 bit)"=w371) -> ("VISA resource name out"=w373:refnum<visa-resource-name>, "error out"=w372:errorcluster)  [unwired: 8 in]
                  }
                  frame #1 {
                    n234 = while {
                      tunnel: w380 -> [w383]
                      tunnel: w379 -> [w382]
                      stop <- w381 stop-if-true
                      n235 = stacked-sequence {
                        tunnel: w383 -> [_ w421]
                        tunnel: w382 -> [_ w420]
                        tunnel: [_ w414] -> w381
                        frame #0 {
                          n236 = disable-structure shown="Enabled" {
                            frame Disabled {
                              n237 = stacked-sequence {
                                frame #0 {
                                n238 = Wait (ms)(milliseconds to wait=u32 500) -> ()  [unwired: 1 out]
                                }
                                frame #1 {
                                # "AMOSTRAGEM (1 VALOR)"
                                n239 = call "Connect_To_Meter.vi"("Location of FieldMax2Lib.dll in"="Location of FieldMax2Lib.dll in 7") -> ("Meter Serial Number"=→"Meter Serial Number 7":string, "Meter ID out"=w394:i32, "Location of FieldMax2Lib.dll out"=w393:path)  [unwired: 6 in]
                                n240 = dll-call lib="C:/Windows/System32/FieldMax2Lib.dll" fn="fm2LibSync" label="Sync"(path in=w393, "h"=w394) -> (path out=w395:path, "h"=w396:i32)  [unwired: 3 in, 1 out]
                                n241 = Initialize Array(u8 0 ("element"), 64 ("dimension size")) -> (w387:u8[])
                                n242 = while {
                                tunnel: w396 -> [w398]
                                tunnel: w387 -> [w404]
                                tunnel: i16 8 ("count") -> [w403]
                                tunnel: [w400] -> w391
                                tunnel: w395 -> [w405]
                                tunnel: [w399] -> w392
                                stop <- w397 stop-if-true
                                n243 = dll-call lib="C:/Windows/System32/FieldMax2Lib.dll" fn="fm2LibGetData" label="Get Data"(path in=w405, "h"=w398, "returnBuffer"=w404, "count"=w403) -> (path out=w399:path, "h"=w400:i32, "returnBuffer"=w401:u8[], "count"=w402:i16)  [unwired: 3 in, 1 out]
                                n244 = Not Equal To 0?(x=w402) -> (x != 0?=w406:bool)
                                n245 = call "Utility - Bytes to Values.vi"("DataBuffer"=w401) -> ("Measurement Value"=w407:sgl)  [unwired: 9 in, 1 out]
                                n246 = Wait (ms)(milliseconds to wait=u32 1000) -> ()  [unwired: 1 out]
                                n247 = case shown="True" w406 {
                                tunnel: w407 -> [_ w411]
                                tunnel: [FALSE TRUE] -> w397
                                frame False {
                                }
                                frame True {
                                n248 = local write "Measurement\n (W)"(w411) -> ()
                                }
                                }
                                }
                                n249 = call "Disconnect_From_Meter.vi"("Location of FieldMax2Lib.dll in"=w392, "Meter ID in"=w391) -> ()  [unwired: 7 in, 2 out]
                                }
                              }
                            }
                            frame Enabled {
                              n250 = flat-sequence {
                                frame #0 {
                                n251 = Wait (ms)(milliseconds to wait=u32 500) -> ()  [unwired: 1 out]
                                }
                                frame #1 {
                                n252 = local write "Measurement\n (W)"(0.145 ("Measurement")) -> ()
                                }
                              }
                            }
                          }
                        }
                        frame #1 {
                          n253 = local read "Measurement\n (W)"() -> (w419:dbl)
                          n254 = local read "Setpoint (W)"() -> (w418:dbl)
                          n255 = Subtract(x=w418, y=w419) -> (x-y=w417:dbl)
                          n256 = Less?(x=w417, y=0.0004) -> (x < y?=w415:bool)
                          n257 = case shown="True" w415 {
                            tunnel: w421 -> [w428 _]
                            tunnel: w420 -> [w422 _]
                            tunnel: [FALSE TRUE] -> w414
                            frame False {
                              # "AJUSTE FINO"
                              n258 = local read "Measurement\n (W)"() -> (w425:dbl)
                              n259 = local read "Setpoint (W)"() -> (w424:dbl)
                              n260 = local write "Erro comando PIC"(w422) -> ()
                              n261 = local write "Motor Disco"(TRUE) -> ()
                              n262 = Greater?(x=w424, y=w425) -> (0:w427:bool)
                              n263 = case shown="False" w427 {
                                tunnel: w424 -> [w433 _]
                                tunnel: w425 -> [w432 _]
                                tunnel: w428 -> [w430 w447]
                                tunnel: w422 -> [w429 w446]
                                frame False {
                                n264 = Equal?(x=w433, y=w432) -> (x = y?=w431:bool)
                                n265 = case shown="False" w431 {
                                tunnel: w430 -> [w436 w442]
                                tunnel: w429 -> [w435 w441]
                                frame False {
                                n266 = VISA Write(VISA resource name=w436, write buffer="D0003OK", error in (no error)=w435) -> (return count=w437:u32, error out=w434:errorcluster)  [unwired: 1 out]
                                n267 = local write "Erro comando PIC"(w434) -> ()
                                n268 = local write "return count"(w437) -> ()
                                }
                                frame True {
                                n269 = VISA Write(VISA resource name=w442, write buffer="S0000OK", error in (no error)=w441) -> (VISA resource name out=w440:refnum<visa-resource-name>, return count=w443:u32, error out=w439:errorcluster)
                                n270 = local write "return count"(w443) -> ()
                                n271 = local write "Erro comando PIC"(w439) -> ()
                                n272 = VISA Close(VISA resource name=w440, error in (no error)=w439) -> ()  [unwired: 1 out]
                                }
                                }
                                }
                                frame True {
                                n273 = VISA Write(VISA resource name=w447, write buffer="I0003OK", error in (no error)=w446) -> (return count=w448:u32, error out=w445:errorcluster)  [unwired: 1 out]
                                n274 = local write "Erro comando PIC"(w445) -> ()
                                n275 = local write "return count"(w448) -> ()
                                }
                              }
                            }
                            frame True {
                            }
                          }
                        }
                      }
                    }
                  }
                }
              }
              frame #5 {
                n276 = stacked-sequence {
                  frame #0 {
                    n277 = Wait (ms)(milliseconds to wait=u32 500) -> ()  [unwired: 1 out]
                  }
                  frame #1 {
                    n278 = disable-structure shown="Enabled" {
                      frame Disabled {
                        # "AMOSTRAGEM (1 VALOR)"
                        n279 = call "Connect_To_Meter.vi"("Location of FieldMax2Lib.dll in"="Location of FieldMax2Lib.dll in 8") -> ("Meter Serial Number"=→"Meter Serial Number 8":string, "Meter ID out"=w461:i32, "Location of FieldMax2Lib.dll out"=w460:path)  [unwired: 6 in]
                        n280 = dll-call lib="C:/Windows/System32/FieldMax2Lib.dll" fn="fm2LibSync" label="Sync"(path in=w460, "h"=w461) -> (path out=w462:path, "h"=w463:i32)  [unwired: 3 in, 1 out]
                        n281 = Initialize Array(u8 0 ("element"), 64 ("dimension size")) -> (w454:u8[])
                        n282 = while {
                          tunnel: w463 -> [w465]
                          tunnel: w454 -> [w471]
                          tunnel: i16 8 ("count") -> [w470]
                          tunnel: [w467] -> w458
                          tunnel: w462 -> [w472]
                          tunnel: [w466] -> w459
                          stop <- w464 stop-if-true
                          n283 = dll-call lib="C:/Windows/System32/FieldMax2Lib.dll" fn="fm2LibGetData" label="Get Data"(path in=w472, "h"=w465, "returnBuffer"=w471, "count"=w470) -> (path out=w466:path, "h"=w467:i32, "returnBuffer"=w468:u8[], "count"=w469:i16)  [unwired: 3 in, 1 out]
                          n284 = Not Equal To 0?(x=w469) -> (x != 0?=w473:bool)
                          n285 = call "Utility - Bytes to Values.vi"("DataBuffer"=w468) -> ("Measurement Value"=w474:sgl)  [unwired: 9 in, 1 out]
                          n286 = Wait (ms)(milliseconds to wait=u32 1000) -> ()  [unwired: 1 out]
                          n287 = case shown="True" w473 {
                            tunnel: w474 -> [_ w478]
                            tunnel: [FALSE TRUE] -> w464
                            frame False {
                            }
                            frame True {
                              n288 = local write "Measurement\n (W)"(w478) -> ()
                            }
                          }
                        }
                        n289 = call "Disconnect_From_Meter.vi"("Location of FieldMax2Lib.dll in"=w459, "Meter ID in"=w458) -> ()  [unwired: 7 in, 2 out]
                      }
                      frame Enabled {
                        n290 = local write "Measurement\n (W)"(0.1159) -> ()
                      }
                    }
                  }
                  frame #2 {
                    n291 = flat-sequence {
                      frame #0 {
                        n292 = local read "Measurement\n (W)"() -> (w483:dbl)
                        n293 = Number To Fractional String(number=w483, precision (6)=i16 4) -> (F-format string=w484:string)  [unwired: 2 in]
                        n294 = Scan From String(format string="%6.4f", input string=w484) -> (output 1=w480:dbl)  [unwired: 3 in, 3 out]
                        n295 = Format Into String(format string="%6.4f", w480) -> (resulting string=w481:string)  [unwired: 2 in, 1 out]
                        n296 = local write "Resulting string (W)"(w481) -> ()
                      }
                      frame #1 {
                        n297 = local read "Resulting string (W)"() -> (w489:string)
                        n298 = Concatenate Strings("Potencia_ajustada:", w489) -> (w487:string)
                        n299 = local write "Resulting string (W)"(w487) -> ()
                      }
                    }
                  }
                }
              }
              frame #6 {
                n300 = flat-sequence {
                  tunnel: [w500] -> w497
                  tunnel: [w498] -> w496
                  tunnel: w497 -> [w509]
                  tunnel: w496 -> [w508]
                  tunnel: [w507] -> w491
                  tunnel: [w506] -> w490
                  tunnel: w491 -> [w517]
                  tunnel: w490 -> [w516]
                  tunnel: [w515] -> w495
                  tunnel: [w514] -> w493
                  tunnel: w495 -> [w524]
                  tunnel: [w524] -> w494
                  tunnel: w493 -> [w523]
                  tunnel: [w523] -> w492
                  tunnel: w494 -> [w528]
                  tunnel: w492 -> [w527]
                  frame #0 {
                    w499 = u16 10 items=["1.0"=10, "1.5"=15, "2.0"=20] ("stop bits (10: 1 bit)")
                    (unwired) u8 13 ("termination char\n(0xA = '\\n' = LF)")
                    (unwired) u16 10 ("data bits (8)")
                    # "CONFIGURAÇÃO COMUNICAÇÃO PIC"
                    n301 = local read "COM PIC"() -> (w505:refnum<visa-resource-name>)
                    n302 = call-poly "VISA Configure Serial Port"("VISA resource name"=w505, "timeout (10sec)"=u32 120000, "Enable Termination\nChar (T)"=TRUE, "baud rate (9600)"=u32 9600, "parity (0:none)"=enum16{"None", "Odd", "Even", "Mark", "Space"}."None", "stop bits (10: 1 bit)"=w499) -> ("VISA resource name out"=w500:refnum<visa-resource-name>, "error out"=w498:errorcluster)  [unwired: 8 in]
                    n303 = local write "Erro comando PIC"(w498) -> ()
                  }
                  frame #1 {
                    # "FECHAMENTO OBTURADOR"
                    n304 = local write "Shutter ON (Verde)/ OFF (Vermelho)"(TRUE ("Inicia Controle")) -> ()
                    n305 = VISA Write(VISA resource name=w509, write buffer="F0000OK", error in (no error)=w508) -> (VISA resource name out=w507:refnum<visa-resource-name>, return count=w513:u32, error out=w506:errorcluster)
                    n306 = local write "return count"(w513) -> ()
                    n307 = local write "Motor Disco"(FALSE) -> ()
                    n308 = local write "Erro comando PIC"(w506) -> ()
                  }
                  frame #2 {
                    # "RETIRADA DO SENSOR"
                    n309 = local write "Shutter ON (Verde)/ OFF (Vermelho)"(TRUE) -> ()
                    n310 = VISA Write(VISA resource name=w517, write buffer="R0000OK", error in (no error)=w516) -> (VISA resource name out=w515:refnum<visa-resource-name>, return count=w518:u32, error out=w514:errorcluster)
                    n311 = local write "return count"(w518) -> ()
                    n312 = local write "Erro comando PIC"(w514) -> ()
                    n313 = local write "Motor Sensor"(TRUE) -> ()
                  }
                  frame #3 {
                    n314 = Wait (ms)(milliseconds to wait=u32 4000) -> ()  [unwired: 1 out]
                  }
                  frame #4 {
                    # "ABERTURA DO OBTURADOR"
                    n315 = local write "Shutter ON (Verde)/ OFF (Vermelho)"(FALSE) -> ()
                    n316 = local write "Motor Sensor"(FALSE) -> ()
                    n317 = VISA Write(VISA resource name=w528, write buffer="F0000OK", error in (no error)=w527) -> (VISA resource name out=w526:refnum<visa-resource-name>, return count=w533:u32, error out=w525:errorcluster)
                    n318 = local write "return count"(w533) -> ()
                    n319 = property on="Setpoint (W)" class="DigNum (strict)"("DisabledEnum"=T2."Enabled" ("Disabled")) -> ()  [unwired: 2 in, 2 out]
                    n320 = VISA Close(VISA resource name=w526, error in (no error)=w525) -> ()  [unwired: 1 out]
                  }
                }
              }
              frame #7 {
                # "potencia_ajustada:0,0000(24caracteres)"
                # "AVISO AO USUÁRIO DE POTÊNCIA AJUSTADA"
                n321 = flat-sequence {
                  frame #0 {
                    n322 = while {
                      stop <- w535 stop-if-true
                      n323 = local read "Resulting string (W)"() -> (w537:string)
                      n324 = One Button Dialog(message=w537, button name ("OK")="Massa!") -> (true=w535:bool)
                    }
                  }
                  frame #1 {
                    n325 = Wait (ms)(milliseconds to wait=u32 3000) -> ()  [unwired: 1 out]
                  }
                }
              }
            }
          }
          frame "Ajuste de Potência" {
            n326 = stacked-sequence {
              tunnel: [_ _ _ _ _ _ TCC_01_02_15."Eventos" ("States")] -> w539
              frame #0 {
                # "CONFERIR REGISTRO SETPONT, VALOR HORARIO E DATA"
                n327 = local read "Setpoint (W)"() -> (w544:dbl)
                n328 = call <vilib>:"Application Directory.vi"() -> ("Application Directory"=w551:path)
                n329 = Path To String(path=w551) -> (string=w549:string)
                n330 = Concatenate Strings(w549, "\\" ("string"), "Config.ini" ("replace string (\"\")")) -> (w550:string)
                n331 = Build Array(w544) -> (w547:dbl[])
                n332 = String To Path(string=w550) -> (path=w548:path)
                n333 = call-poly <vilib>:"Write To Spreadsheet File.vi"("append to file? (new file:F)"=TRUE, "1D data"=w547, "file path (dialog if empty)"=w548) -> ()  [unwired: 5 in, 1 out]
                n334 = local write "Shutter ON (Verde)/ OFF (Vermelho)"(TRUE) -> ()
                n335 = local write "Motor Sensor"(FALSE) -> ()
                n336 = local write "Motor Disco"(FALSE) -> ()
              }
              frame #1 {
                n337 = flat-sequence {
                  tunnel: [w571] -> w563
                  tunnel: [w569] -> w561
                  tunnel: w563 -> [w582]
                  tunnel: [w582] -> w562
                  tunnel: w561 -> [w581]
                  tunnel: [w581] -> w560
                  tunnel: w562 -> [w585]
                  tunnel: w560 -> [w586]
                  tunnel: [w584] -> w555
                  tunnel: [w583] -> w553
                  tunnel: w555 -> [w594]
                  tunnel: [w594] -> w554
                  tunnel: w553 -> [w593]
                  tunnel: [w593] -> w552
                  tunnel: w554 -> [w598]
                  tunnel: w552 -> [w597]
                  tunnel: [w596] -> w559
                  tunnel: [w595] -> w557
                  tunnel: w559 -> [w605]
                  tunnel: [w605] -> w558
                  tunnel: w557 -> [w604]
                  tunnel: [w604] -> w556
                  tunnel: w558 -> [w609]
                  tunnel: w556 -> [w608]
                  tunnel: [w607] -> w566
                  tunnel: [w606] -> w564
                  tunnel: [w614] -> w567
                  tunnel: w566 -> [w614]
                  tunnel: [w613] -> w565
                  tunnel: w564 -> [w613]
                  tunnel: w567 -> [w617]
                  tunnel: w565 -> [w616]
                  frame #0 {
                    w570 = u16 10 items=["1.0"=10, "1.5"=15, "2.0"=20] ("stop bits (10: 1 bit)")
                    (unwired) u32 120000 ("timeout (10sec)")
                    (unwired) u16 10 ("data bits (8)")
                    # "CONFIGURAÇÃO COMUNICAÇÃO PIC"
                    n338 = local read "COM PIC"() -> (w579:refnum<visa-resource-name>)
                    n339 = local write "Shutter ON (Verde)/ OFF (Vermelho)"(FALSE ("Inicia Controle")) -> ()
                    n340 = local write "Motor Disco"(FALSE) -> ()
                    n341 = local write "Motor Sensor"(FALSE) -> ()
                    n342 = call-poly "VISA Configure Serial Port"("VISA resource name"=w579, "termination char\n(0xA = '\\n' = LF)"=u8 13 ("termination char\n(0xA = '\\n' = LF)"), "Enable Termination\nChar (T)"=TRUE, "baud rate (9600)"=u32 9600, "parity (0:none)"=enum16{"None", "Odd", "Even", "Mark", "Space"}."None", "stop bits (10: 1 bit)"=w570) -> ("VISA resource name out"=w571:refnum<visa-resource-name>, "error out"=w569:errorcluster)  [unwired: 8 in]
                    n343 = local write "Erro comando PIC"(w569) -> ()
                  }
                  frame #1 {
                    n344 = Wait (ms)(milliseconds to wait=500) -> ()  [unwired: 1 out]
                  }
                  frame #2 {
                    # "FECHAMENTO OBTURADOR"
                    n345 = local write "Shutter ON (Verde)/ OFF (Vermelho)"(TRUE) -> ()
                    n346 = VISA Write(VISA resource name=w585, write buffer="F0000OK", error in (no error)=w586) -> (VISA resource name out=w584:refnum<visa-resource-name>, return count=w590:u32, error out=w583:errorcluster)
                    n347 = local write "return count"(w590) -> ()
                    n348 = local write "Motor Sensor"(FALSE) -> ()
                    n349 = local write "Motor Disco"(FALSE) -> ()
                    n350 = local write "Erro comando PIC"(w583) -> ()
                  }
                  frame #3 {
                    n351 = Wait (ms)(milliseconds to wait=u32 3000) -> ()  [unwired: 1 out]
                  }
                  frame #4 {
                    # "POSICIONAMENTO SENSOR"
                    n352 = local write "Shutter ON (Verde)/ OFF (Vermelho)"(TRUE) -> ()
                    n353 = VISA Write(VISA resource name=w598, write buffer="P0000OK", error in (no error)=w597) -> (VISA resource name out=w596:refnum<visa-resource-name>, return count=w602:u32, error out=w595:errorcluster)
                    n354 = local write "Erro comando PIC"(w595) -> ()
                    n355 = local write "return count"(w602) -> ()
                    n356 = local write "Motor Sensor"(TRUE) -> ()
                  }
                  frame #5 {
                    n357 = Wait (ms)(milliseconds to wait=u32 4000) -> ()  [unwired: 1 out]
                  }
                  frame #6 {
                    # "ABERTURA DO OBTURADOR E HOLD-OFF\n ESTABILIAZAÇÃO SENSOR"
                    n358 = local write "Shutter ON (Verde)/ OFF (Vermelho)"(FALSE) -> ()
                    n359 = VISA Write(VISA resource name=w609, write buffer="A0000OK", error in (no error)=w608) -> (VISA resource name out=w607:refnum<visa-resource-name>, return count=w612:u32, error out=w606:errorcluster)
                    n360 = local write "return count"(w612) -> ()
                    n361 = local write "Erro comando PIC"(w606) -> ()
                  }
                  frame #7 {
                    # "Atraso após\nestabilidade\ntérmica"
                    n362 = Wait (ms)(milliseconds to wait=u32 3000) -> ()  [unwired: 1 out]
                  }
                  frame #8 {
                    n363 = VISA Close(VISA resource name=w617, error in (no error)=w616) -> ()  [unwired: 1 out]
                  }
                }
                n364 = property on="Setpoint (W)" class="DigNum (strict)"("DisabledEnum"=T2."Disabled" ("Disabled")) -> ()  [unwired: 2 in, 2 out]
              }
              frame #2 {
                n365 = while {
                  i -> [w618]
                  stop <- w619 stop-if-true
                  n366 = stacked-sequence {
                    tunnel: [_ _ w844] -> w619
                    frame #0 {
                      n367 = while {
                        stop <- w620 stop-if-true
                        n368 = flat-sequence {
                          tunnel: [w662] -> w620
                          frame #0 {
                            n369 = disable-structure shown="Enabled" {
                              frame Enabled {
                                # "AMOSTRAGEM INICIAL (20 VALORES)"
                                n370 = call "Connect_To_Meter.vi"("Location of FieldMax2Lib.dll in"="Location of FieldMax2Lib.dll in 3") -> ("Meter Serial Number"=→"Meter Serial Number 3":string, "Meter ID out"=w623:i32, "Location of FieldMax2Lib.dll out"=w624:path)  [unwired: 6 in]
                                n371 = dll-call lib="C:/Windows/System32/FieldMax2Lib.dll" fn="fm2LibSync" label="Sync"(path in=w624, "h"=w623) -> (path out=w622:path, "h"=w621:i32)  [unwired: 3 in, 1 out]
                                n372 = Initialize Array(u8 0 ("element"), 64 ("dimension size")) -> (w630:u8[])
                                n373 = for {
                                N: 21 -> [_]
                                tunnel: w621 -> [w639]
                                tunnel: w630 -> [w645]
                                tunnel: i16 8 ("count") -> [w644]
                                tunnel: [w641] -> w626
                                tunnel: w622 -> [w646]
                                tunnel: [w640] -> w625
                                shift-right: [w636] -> w634
                                shift-left: sgl[] [] -> [w637]
                                i -> [w638]
                                n374 = dll-call lib="C:/Windows/System32/FieldMax2Lib.dll" fn="fm2LibGetData" label="Get Data"(path in=w646, "h"=w639, "returnBuffer"=w645, "count"=w644) -> (path out=w640:path, "h"=w641:i32, "returnBuffer"=w642:u8[], "count"=w643:i16)  [unwired: 3 in, 1 out]
                                n375 = Not Equal To 0?(x=w643) -> (x != 0?=w647:bool)
                                n376 = call "Utility - Bytes to Values.vi"("DataBuffer"=w642) -> ("Measurement Value"=w648:sgl)  [unwired: 9 in, 1 out]
                                n377 = Wait (ms)(milliseconds to wait=u32 1000) -> ()  [unwired: 1 out]
                                n378 = case shown="False" w647 {
                                tunnel: w648 -> [w651 w652]
                                tunnel: [w651 w652] -> _
                                tunnel: w637 -> [w650 w654]
                                tunnel: [w650 w653] -> w636
                                frame False {
                                (unwired) FALSE
                                }
                                frame True {
                                n379 = local write "Measurement\n (W)"(w652) -> ()
                                n380 = Build Array (concatenate)(w654, w652) -> (w653:sgl[])
                                }
                                }
                                "Loop" <- w638
                                }
                                "initialized array" <- w634
                                n381 = call "Disconnect_From_Meter.vi"("Location of FieldMax2Lib.dll in"=w625, "Meter ID in"=w626) -> ()  [unwired: 7 in, 2 out]
                              }
                              frame Disabled {
                                n382 = Wait (ms)(milliseconds to wait=u32 500) -> ()  [unwired: 1 out]
                                n383 = local write "Medida (W)"(0.105 ("Measurement")) -> ()
                              }
                            }
                          }
                          frame #1 {
                            # "CALCULO DO VALOR MEDIO DA BATERIA DE\nVALORES E SEU DESVIO PADRÃO (VALIDAÇÃO)"
                            n384 = disable-structure shown="Enabled" {
                              frame Enabled {
                                n385 = local read "initialized array"() -> (w658:sgl[])
                                n386 = call <vilib>:"Std Deviation and Variance.vi"("X"=w658, "Weighting (Sample)"=enum16{"Sample", "Population"}."Population") -> ("mean"=w661:dbl, "standard deviation"=w660:dbl)  [unwired: 1 out]
                                n387 = local write "Medida (W)"(w661) -> ()
                                n388 = local write "Desv.Padrão"(w660) -> ()
                              }
                              frame Disabled {
                              }
                            }
                            n389 = Wait (ms)(milliseconds to wait=u32 2000) -> ()  [unwired: 1 out]
                          }
                          frame #2 {
                            n390 = local read "Desv.Padrão"() -> (w663:dbl)
                            n391 = Less?(x=w663, y=0.0004) -> (x < y?=w662:bool)
                          }
                        }
                      }
                    }
                    frame #1 {
                      n392 = local read "i"() -> (w667:i32)
                      n393 = Greater?(x=w667, y=1) -> (0:w665:bool)
                      n394 = case shown="True" w665 {
                        frame False {
                          # "TRUNCAMENTO DA DIFERENÇA \nPARA RESOLUÇÃO MÁXIMA DO\nSISTEMA"
                          # "Maxima potência\n0.009(min)W"
                          # "Diferença truncada\n(DBL)"
                          n395 = local read "Setpoint (W)"() -> (w677:dbl)
                          n396 = local read "Medida (W)"() -> (w676:dbl)
                          n397 = Subtract(x=w677, y=w676) -> (x-y=w670:dbl)
                          n398 = Number To Fractional String(number=w670, precision (6)=i16 4) -> (F-format string=w673:string)  [unwired: 2 in]
                          n399 = Scan From String(format string="%7.4f", input string=w673) -> (output 1=w674:dbl)  [unwired: 3 in, 3 out]
                          n400 = Divide(x=w674, y="Potência max Laser") -> (x/y=w669:dbl)
                          n401 = flat-sequence {
                            tunnel: w669 -> [w683]
                            tunnel: [w683] -> w681
                            tunnel: w681 -> [w695]
                            tunnel: [w695] -> w680
                            tunnel: [w689] -> w679
                            tunnel: [w687] -> w678
                            tunnel: w680 -> [w698]
                            tunnel: w679 -> [w697]
                            tunnel: w678 -> [w696]
                            frame #0 {
                              # "CONVERSÃO DA DIFERENÇA\nTRUNCADA PARA NÚMERO\nDE PASSOS"
                              # "vai alterar devido a diferença da volta \ndo eixo do motor para a do disco"
                              n402 = Absolute Value(x=w683) -> (abs(x)=w682:dbl)
                              "Diferença em %" <- w682
                              n403 = Divide(x=w682, y=0.0024218) -> (x/y=w685:dbl)
                              n404 = Round To Nearest(number=w685) -> (nearest integer value=w686:dbl)
                              n405 = local write "Quantidade de Passos"(w686) -> ()
                            }
                            frame #1 {
                              w688 = u16 10 items=["1.0"=10, "1.5"=15, "2.0"=20] ("stop bits (10: 1 bit)")
                              (unwired) u16 10 ("data bits (8)")
                              # "CONFIGURAÇÃO \nCOM PIC"
                              n406 = local read "COM PIC"() -> (w690:refnum<visa-resource-name>)
                              n407 = call-poly "VISA Configure Serial Port"("VISA resource name"=w690, "timeout (10sec)"=u32 120000, "Enable Termination\nChar (T)"=TRUE, "baud rate (9600)"=u32 9600, "parity (0:none)"=enum16{"None", "Odd", "Even", "Mark", "Space"}."None", "stop bits (10: 1 bit)"=w688) -> ("VISA resource name out"=w689:refnum<visa-resource-name>, "error out"=w687:errorcluster)  [unwired: 8 in]
                              n408 = local write "Erro comando PIC"(w687) -> ()
                            }
                            frame #2 {
                              # "AJUSTE GROSSO"
                              n409 = Greater Than 0?(x=w698) -> (x > 0?=w699:bool)
                              n410 = case shown="True" w699 {
                                tunnel: w697 -> [w703 w727]
                                tunnel: w696 -> [w702 w728]
                                frame False {
                                n411 = stacked-sequence {
                                tunnel: [_ _ w724] -> w705
                                frame #0 {
                                n412 = local read "Quantidade de Passos"() -> (w706:sgl)
                                n413 = Format Into String(format string="%d", w706) -> (resulting string=w708:string)  [unwired: 2 in, 1 out]
                                n414 = String Length(string=w708) -> (length=w709:i32)
                                n415 = case shown="1, Default" w709 {
                                tunnel: w708 -> [w711 w714 w716 w719]
                                frame 1, Default {
                                n416 = Concatenate Strings("000" ("string"), w711) -> (w712:string)
                                n417 = local write "N_passos string"(w712) -> ()
                                }
                                frame 2 {
                                n418 = Concatenate Strings("00" ("string"), w714) -> (w713:string)
                                n419 = local write "N_passos string"(w713) -> ()
                                }
                                frame 3 {
                                n420 = Concatenate Strings("0" ("string"), w716) -> (w717:string)
                                n421 = local write "N_passos string"(w717) -> ()
                                }
                                frame 4 {
                                n422 = local write "N_passos string"(w719) -> ()
                                }
                                }
                                }
                                frame #1 {
                                # "adicionar letra"
                                n423 = local read "N_passos string"() -> (w721:string)
                                n424 = Concatenate Strings("D" ("string"), w721, "OK" ("string")) -> (w723:string)
                                n425 = local write "N_passos string"(w723) -> ()
                                }
                                frame #2 {
                                n426 = local read "N_passos string"() -> (w724:string)
                                }
                                }
                                n427 = VISA Write(VISA resource name=w703, write buffer=w705, error in (no error)=w702) -> (VISA resource name out=w701:refnum<visa-resource-name>, return count=w704:u32, error out=w700:errorcluster)
                                n428 = local write "Erro comando PIC"(w700) -> ()
                                n429 = local write "return count"(w704) -> ()
                                n430 = VISA Close(VISA resource name=w701, error in (no error)=w700) -> ()  [unwired: 1 out]
                                }
                                frame True {
                                n431 = stacked-sequence {
                                tunnel: [_ _ w749] -> w730
                                frame #0 {
                                n432 = local read "Quantidade de Passos"() -> (w731:sgl)
                                n433 = Format Into String(format string="%d", w731) -> (resulting string=w733:string)  [unwired: 2 in, 1 out]
                                n434 = String Length(string=w733) -> (length=w734:i32)
                                n435 = case shown="3" w734 {
                                tunnel: w733 -> [w735 w739 w741 w744]
                                frame 1, Default {
                                n436 = Concatenate Strings("000" ("string"), w735) -> (w737:string)
                                n437 = local write "N_passos string"(w737) -> ()
                                }
                                frame 2 {
                                n438 = Concatenate Strings("00" ("string"), w739) -> (w738:string)
                                n439 = local write "N_passos string"(w738) -> ()
                                }
                                frame 3 {
                                n440 = Concatenate Strings("0" ("string"), w741) -> (w742:string)
                                n441 = local write "N_passos string"(w742) -> ()
                                }
                                frame 4 {
                                n442 = local write "N_passos string"(w744) -> ()
                                }
                                }
                                }
                                frame #1 {
                                n443 = local read "N_passos string"() -> (w746:string)
                                n444 = Concatenate Strings("I" ("string"), w746, "OK" ("string")) -> (w748:string)
                                n445 = local write "N_passos string"(w748) -> ()
                                }
                                frame #2 {
                                n446 = local read "N_passos string"() -> (w749:string)
                                }
                                }
                                n447 = VISA Write(VISA resource name=w727, write buffer=w730, error in (no error)=w728) -> (VISA resource name out=w726:refnum<visa-resource-name>, return count=w729:u32, error out=w725:errorcluster)
                                n448 = local write "Erro comando PIC"(w725) -> ()
                                n449 = local write "return count"(w729) -> ()
                                n450 = VISA Close(VISA resource name=w726, error in (no error)=w725) -> ()  [unwired: 1 out]
                                }
                              }
                            }
                            frame #3 {
                              n451 = local read "Quantidade de Passos"() -> (→"Quantidade de Passos N-1":sgl)
                              n452 = local read "Medida (W)"() -> (→"Medida N-1 (W)":dbl)
                            }
                            frame #4 {
                              n453 = Wait (ms)(milliseconds to wait=8000) -> ()  [unwired: 1 out]
                            }
                          }
                          n454 = local write "Motor Disco"(TRUE) -> ()
                        }
                        frame True {
                          n455 = stacked-sequence {
                            frame #0 {
                              n456 = flat-sequence {
                                frame #0 {
                                n457 = local read "Medida N-1 (W)"() -> (w754:dbl)
                                n458 = local read "Medida (W)"() -> (w755:dbl)
                                n459 = Subtract(x=w754, y=w755) -> (x-y=→"DeltaP":dbl)
                                }
                                frame #1 {
                                n460 = local read "Quantidade de Passos N-1"() -> (w758:sgl)
                                n461 = local read "DeltaP"() -> (w757:dbl)
                                n462 = Divide(x=w757, y=w758) -> (x/y=→"Coeficiente novo":dbl)
                                }
                                frame #2 {
                                n463 = local read "Quantidade de Passos N-1"() -> (w760:sgl)
                                n464 = local read "Medida (W)"() -> (w759:dbl)
                                n465 = local write "Medida N-1 (W)"(w759) -> ()
                                n466 = local write "Quantidade de Passos"(w760) -> ()
                                }
                              }
                            }
                            frame #1 {
                              # "TRUNCAMENTO DA DIFERENÇA \nPARA RESOLUÇÃO MÁXIMA DO\nSISTEMA"
                              # "Maxima potência\n0.009(min)W"
                              # "Diferença truncada\n(DBL)"
                              n467 = local read "Setpoint (W)"() -> (w769:dbl)
                              n468 = local read "Medida (W)"() -> (w768:dbl)
                              n469 = local read "Potência max Laser"() -> (w770:dbl)
                              n470 = Subtract(x=w769, y=w768) -> (x-y=w762:dbl)
                              n471 = Number To Fractional String(number=w762, precision (6)=i16 4) -> (F-format string=w765:string)  [unwired: 2 in]
                              n472 = Scan From String(format string="%7.4f", input string=w765) -> (output 1=w766:dbl)  [unwired: 3 in, 3 out]
                              n473 = Divide(x=w766, y=w770) -> (x/y=w761:dbl)
                              n474 = flat-sequence {
                                tunnel: w761 -> [w777]
                                tunnel: [w777] -> w774
                                tunnel: w774 -> [w788]
                                tunnel: [w788] -> w773
                                tunnel: [w782] -> w772
                                tunnel: [w780] -> w771
                                tunnel: w773 -> [w791]
                                tunnel: w772 -> [w790]
                                tunnel: w771 -> [w789]
                                frame #0 {
                                # "CONVERSÃO DA DIFERENÇA\nTRUNCADA PARA NÚMERO\nDE PASSOS"
                                # "vai alterar devido a diferença da volta \ndo eixo do motor para a do disco"
                                n475 = local read "Coeficiente novo"() -> (w776:dbl)
                                n476 = Absolute Value(x=w777) -> (abs(x)=w775:dbl)
                                n477 = local write "Diferença em %"(w775) -> ()
                                n478 = Divide(x=w775, y=w776) -> (x/y=w778:dbl)
                                n479 = Round To Nearest(number=w778) -> (nearest integer value=w779:dbl)
                                n480 = local write "Quantidade de Passos"(w779) -> ()
                                }
                                frame #1 {
                                w781 = u16 10 items=["1.0"=10, "1.5"=15, "2.0"=20] ("stop bits (10: 1 bit)")
                                (unwired) u16 10 ("data bits (8)")
                                # "CONFIGURAÇÃO \nCOM PIC"
                                n481 = local read "COM PIC"() -> (w783:refnum<visa-resource-name>)
                                n482 = call-poly "VISA Configure Serial Port"("VISA resource name"=w783, "timeout (10sec)"=u32 120000, "Enable Termination\nChar (T)"=TRUE, "baud rate (9600)"=u32 9600, "parity (0:none)"=enum16{"None", "Odd", "Even", "Mark", "Space"}."None", "stop bits (10: 1 bit)"=w781) -> ("VISA resource name out"=w782:refnum<visa-resource-name>, "error out"=w780:errorcluster)  [unwired: 8 in]
                                n483 = local write "Erro comando PIC"(w780) -> ()
                                }
                                frame #2 {
                                # "AJUSTE GROSSO"
                                n484 = Greater Than 0?(x=w791) -> (x > 0?=w792:bool)
                                n485 = case shown="True" w792 {
                                tunnel: w790 -> [w796 w820]
                                tunnel: w789 -> [w795 w821]
                                frame False {
                                n486 = stacked-sequence {
                                tunnel: [_ _ w817] -> w798
                                frame #0 {
                                n487 = local read "Quantidade de Passos"() -> (w799:sgl)
                                n488 = Format Into String(format string="%d", w799) -> (resulting string=w801:string)  [unwired: 2 in, 1 out]
                                n489 = String Length(string=w801) -> (length=w802:i32)
                                n490 = case shown="1, Default" w802 {
                                tunnel: w801 -> [w804 w807 w809 w812]
                                frame 1, Default {
                                n491 = Concatenate Strings("000" ("string"), w804) -> (w805:string)
                                n492 = local write "N_passos string"(w805) -> ()
                                }
                                frame 2 {
                                n493 = Concatenate Strings("00" ("string"), w807) -> (w806:string)
                                n494 = local write "N_passos string"(w806) -> ()
                                }
                                frame 3 {
                                n495 = Concatenate Strings("0" ("string"), w809) -> (w810:string)
                                n496 = local write "N_passos string"(w810) -> ()
                                }
                                frame 4 {
                                n497 = local write "N_passos string"(w812) -> ()
                                }
                                }
                                }
                                frame #1 {
                                # "adicionar letra"
                                n498 = local read "N_passos string"() -> (w814:string)
                                n499 = Concatenate Strings("D" ("string"), w814, "OK" ("string")) -> (w816:string)
                                n500 = local write "N_passos string"(w816) -> ()
                                }
                                frame #2 {
                                n501 = local read "N_passos string"() -> (w817:string)
                                }
                                }
                                n502 = VISA Write(VISA resource name=w796, write buffer=w798, error in (no error)=w795) -> (VISA resource name out=w794:refnum<visa-resource-name>, return count=w797:u32, error out=w793:errorcluster)
                                n503 = local write "Erro comando PIC"(w793) -> ()
                                n504 = local write "return count"(w797) -> ()
                                n505 = VISA Close(VISA resource name=w794, error in (no error)=w793) -> ()  [unwired: 1 out]
                                }
                                frame True {
                                n506 = stacked-sequence {
                                tunnel: [_ _ w842] -> w823
                                frame #0 {
                                n507 = local read "Quantidade de Passos"() -> (w824:sgl)
                                n508 = Format Into String(format string="%d", w824) -> (resulting string=w826:string)  [unwired: 2 in, 1 out]
                                n509 = String Length(string=w826) -> (length=w827:i32)
                                n510 = case shown="3" w827 {
                                tunnel: w826 -> [w828 w832 w834 w837]
                                frame 1, Default {
                                n511 = Concatenate Strings("000" ("string"), w828) -> (w830:string)
                                n512 = local write "N_passos string"(w830) -> ()
                                }
                                frame 2 {
                                n513 = Concatenate Strings("00" ("string"), w832) -> (w831:string)
                                n514 = local write "N_passos string"(w831) -> ()
                                }
                                frame 3 {
                                n515 = Concatenate Strings("0" ("string"), w834) -> (w835:string)
                                n516 = local write "N_passos string"(w835) -> ()
                                }
                                frame 4 {
                                n517 = local write "N_passos string"(w837) -> ()
                                }
                                }
                                }
                                frame #1 {
                                n518 = local read "N_passos string"() -> (w839:string)
                                n519 = Concatenate Strings("I" ("string"), w839, "OK" ("string")) -> (w841:string)
                                n520 = local write "N_passos string"(w841) -> ()
                                }
                                frame #2 {
                                n521 = local read "N_passos string"() -> (w842:string)
                                }
                                }
                                n522 = VISA Write(VISA resource name=w820, write buffer=w823, error in (no error)=w821) -> (VISA resource name out=w819:refnum<visa-resource-name>, return count=w822:u32, error out=w818:errorcluster)
                                n523 = local write "Erro comando PIC"(w818) -> ()
                                n524 = local write "return count"(w822) -> ()
                                n525 = VISA Close(VISA resource name=w819, error in (no error)=w818) -> ()  [unwired: 1 out]
                                }
                                }
                                }
                                frame #3 {
                                n526 = Wait (ms)(milliseconds to wait=8000) -> ()  [unwired: 1 out]
                                }
                              }
                              n527 = local write "Motor Disco"(TRUE) -> ()
                            }
                          }
                        }
                      }
                    }
                    frame #2 {
                      n528 = local read "Diferença em %"() -> (w845:dbl)
                      n529 = Less?(x=w845, y=0.05) -> (x < y?=w844:bool)
                    }
                  }
                  "i" <- w618
                }
              }
              frame #3 {
                n530 = flat-sequence {
                  tunnel: [w851] -> w848
                  tunnel: [w850] -> w847
                  tunnel: w848 -> [w859]
                  tunnel: w847 -> [w858]
                  frame #0 {
                    w849 = u16 10 items=["1.0"=10, "1.5"=15, "2.0"=20] ("stop bits (10: 1 bit)")
                    (unwired) u8 13 ("termination char\n(0xA = '\\n' = LF)")
                    (unwired) u16 10 ("data bits (8)")
                    # "CONFIGURAÇÃO COMUNICAÇÃO PIC"
                    n531 = local read "COM PIC"() -> (w856:refnum<visa-resource-name>)
                    n532 = call-poly "VISA Configure Serial Port"("VISA resource name"=w856, "timeout (10sec)"=u32 120000, "Enable Termination\nChar (T)"=TRUE, "baud rate (9600)"=u32 9600, "parity (0:none)"=enum16{"None", "Odd", "Even", "Mark", "Space"}."None", "stop bits (10: 1 bit)"=w849) -> ("VISA resource name out"=w851:refnum<visa-resource-name>, "error out"=w850:errorcluster)  [unwired: 8 in]
                  }
                  frame #1 {
                    n533 = while {
                      tunnel: w859 -> [w862]
                      tunnel: w858 -> [w861]
                      stop <- w860 stop-if-true
                      n534 = stacked-sequence {
                        tunnel: w862 -> [_ w901]
                        tunnel: w861 -> [_ w900]
                        tunnel: [_ w895] -> w860
                        frame #0 {
                          n535 = disable-structure shown="Enabled" {
                            frame Enabled {
                              n536 = stacked-sequence {
                                frame #0 {
                                n537 = Wait (ms)(milliseconds to wait=u32 3000) -> ()  [unwired: 1 out]
                                }
                                frame #1 {
                                # "AMOSTRAGEM (1 VALOR)"
                                n538 = call "Connect_To_Meter.vi"("Location of FieldMax2Lib.dll in"="Location of FieldMax2Lib.dll in 4") -> ("Meter Serial Number"=→"Meter Serial Number 4":string, "Meter ID out"=w873:i32, "Location of FieldMax2Lib.dll out"=w872:path)  [unwired: 6 in]
                                n539 = dll-call lib="C:/Windows/System32/FieldMax2Lib.dll" fn="fm2LibSync" label="Sync"(path in=w872, "h"=w873) -> (path out=w874:path, "h"=w875:i32)  [unwired: 3 in, 1 out]
                                n540 = Initialize Array(u8 0 ("element"), 64 ("dimension size")) -> (w866:u8[])
                                n541 = while {
                                tunnel: w875 -> [w877]
                                tunnel: w866 -> [w883]
                                tunnel: i16 8 ("count") -> [w882]
                                tunnel: [w879] -> w870
                                tunnel: w874 -> [w884]
                                tunnel: [w878] -> w871
                                stop <- w876 stop-if-true
                                n542 = dll-call lib="C:/Windows/System32/FieldMax2Lib.dll" fn="fm2LibGetData" label="Get Data"(path in=w884, "h"=w877, "returnBuffer"=w883, "count"=w882) -> (path out=w878:path, "h"=w879:i32, "returnBuffer"=w880:u8[], "count"=w881:i16)  [unwired: 3 in, 1 out]
                                n543 = Not Equal To 0?(x=w881) -> (x != 0?=w885:bool)
                                n544 = call "Utility - Bytes to Values.vi"("DataBuffer"=w880) -> ("Measurement Value"=w886:sgl)  [unwired: 9 in, 1 out]
                                n545 = Wait (ms)(milliseconds to wait=u32 1000) -> ()  [unwired: 1 out]
                                n546 = case shown="True" w885 {
                                tunnel: w886 -> [_ w890]
                                tunnel: [FALSE TRUE] -> w876
                                frame False {
                                }
                                frame True {
                                n547 = local write "Measurement\n (W)"(w890) -> ()
                                }
                                }
                                }
                                n548 = call "Disconnect_From_Meter.vi"("Location of FieldMax2Lib.dll in"=w871, "Meter ID in"=w870) -> ()  [unwired: 7 in, 2 out]
                                }
                              }
                            }
                            frame Disabled {
                              n549 = flat-sequence {
                                frame #0 {
                                n550 = Wait (ms)(milliseconds to wait=u32 500) -> ()  [unwired: 1 out]
                                }
                                frame #1 {
                                n551 = local write "Measurement\n (W)"(0.145 ("Measurement")) -> ()
                                }
                              }
                            }
                          }
                        }
                        frame #1 {
                          n552 = local read "Measurement\n (W)"() -> (w899:dbl)
                          n553 = local read "Setpoint (W)"() -> (w898:dbl)
                          n554 = Subtract(x=w898, y=w899) -> (x-y=w894:dbl)
                          n555 = Absolute Value(x=w894) -> (abs(x)=w893:dbl)
                          n556 = Less?(x=w893, y=0.0004) -> (x < y?=w896:bool)
                          n557 = case shown="False" w896 {
                            tunnel: w901 -> [w908 _]
                            tunnel: w900 -> [w902 _]
                            tunnel: [FALSE TRUE] -> w895
                            frame False {
                              # "AJUSTE FINO"
                              n558 = local read "Measurement\n (W)"() -> (w905:dbl)
                              n559 = local read "Setpoint (W)"() -> (w904:dbl)
                              n560 = local write "Erro comando PIC"(w902) -> ()
                              n561 = local write "Motor Disco"(TRUE) -> ()
                              n562 = Greater?(x=w904, y=w905) -> (0:w907:bool)
                              n563 = case shown="True" w907 {
                                tunnel: w904 -> [w913 _]
                                tunnel: w905 -> [w912 _]
                                tunnel: w908 -> [w910 w927]
                                tunnel: w902 -> [w909 w926]
                                frame False {
                                n564 = Equal?(x=w913, y=w912) -> (x = y?=w911:bool)
                                n565 = case shown="False" w911 {
                                tunnel: w910 -> [w916 w922]
                                tunnel: w909 -> [w915 w921]
                                frame False {
                                n566 = VISA Write(VISA resource name=w916, write buffer="D0001OK", error in (no error)=w915) -> (return count=w917:u32, error out=w914:errorcluster)  [unwired: 1 out]
                                n567 = local write "Erro comando PIC"(w914) -> ()
                                n568 = local write "return count"(w917) -> ()
                                }
                                frame True {
                                n569 = VISA Write(VISA resource name=w922, write buffer="S0000OK", error in (no error)=w921) -> (VISA resource name out=w920:refnum<visa-resource-name>, return count=w923:u32, error out=w919:errorcluster)
                                n570 = local write "return count"(w923) -> ()
                                n571 = local write "Erro comando PIC"(w919) -> ()
                                n572 = VISA Close(VISA resource name=w920, error in (no error)=w919) -> ()  [unwired: 1 out]
                                }
                                }
                                }
                                frame True {
                                n573 = VISA Write(VISA resource name=w927, write buffer="I0001OK", error in (no error)=w926) -> (return count=w928:u32, error out=w925:errorcluster)  [unwired: 1 out]
                                n574 = local write "Erro comando PIC"(w925) -> ()
                                n575 = local write "return count"(w928) -> ()
                                }
                              }
                            }
                            frame True {
                            }
                          }
                        }
                      }
                    }
                    n576 = Wait (ms)(milliseconds to wait=u32 3000) -> ()  [unwired: 1 out]
                  }
                }
              }
              frame #4 {
                n577 = stacked-sequence {
                  frame #0 {
                    n578 = Wait (ms)(milliseconds to wait=u32 500) -> ()  [unwired: 1 out]
                  }
                  frame #1 {
                    n579 = disable-structure shown="Enabled" {
                      frame Enabled {
                        # "AMOSTRAGEM (1 VALOR)"
                        n580 = call "Connect_To_Meter.vi"("Location of FieldMax2Lib.dll in"="Location of FieldMax2Lib.dll in 5") -> ("Meter Serial Number"=→"Meter Serial Number 5":string, "Meter ID out"=w941:i32, "Location of FieldMax2Lib.dll out"=w940:path)  [unwired: 6 in]
                        n581 = dll-call lib="C:/Windows/System32/FieldMax2Lib.dll" fn="fm2LibSync" label="Sync"(path in=w940, "h"=w941) -> (path out=w942:path, "h"=w943:i32)  [unwired: 3 in, 1 out]
                        n582 = Initialize Array(u8 0 ("element"), 64 ("dimension size")) -> (w934:u8[])
                        n583 = while {
                          tunnel: w943 -> [w945]
                          tunnel: w934 -> [w951]
                          tunnel: i16 8 ("count") -> [w950]
                          tunnel: [w947] -> w938
                          tunnel: w942 -> [w952]
                          tunnel: [w946] -> w939
                          stop <- w944 stop-if-true
                          n584 = dll-call lib="C:/Windows/System32/FieldMax2Lib.dll" fn="fm2LibGetData" label="Get Data"(path in=w952, "h"=w945, "returnBuffer"=w951, "count"=w950) -> (path out=w946:path, "h"=w947:i32, "returnBuffer"=w948:u8[], "count"=w949:i16)  [unwired: 3 in, 1 out]
                          n585 = Not Equal To 0?(x=w949) -> (x != 0?=w953:bool)
                          n586 = call "Utility - Bytes to Values.vi"("DataBuffer"=w948) -> ("Measurement Value"=w954:sgl)  [unwired: 9 in, 1 out]
                          n587 = Wait (ms)(milliseconds to wait=u32 1000) -> ()  [unwired: 1 out]
                          n588 = case shown="True" w953 {
                            tunnel: w954 -> [_ w958]
                            tunnel: [FALSE TRUE] -> w944
                            frame False {
                            }
                            frame True {
                              n589 = local write "Measurement\n (W)"(w958) -> ()
                            }
                          }
                        }
                        n590 = call "Disconnect_From_Meter.vi"("Location of FieldMax2Lib.dll in"=w939, "Meter ID in"=w938) -> ()  [unwired: 7 in, 2 out]
                      }
                      frame Disabled {
                        n591 = local write "Measurement\n (W)"(0.1159) -> ()
                      }
                    }
                  }
                  frame #2 {
                    n592 = flat-sequence {
                      frame #0 {
                        n593 = local read "Measurement\n (W)"() -> (w963:dbl)
                        n594 = Number To Fractional String(number=w963, precision (6)=i16 4) -> (F-format string=w964:string)  [unwired: 2 in]
                        n595 = Scan From String(format string="%6.4f", input string=w964) -> (output 1=w960:dbl)  [unwired: 3 in, 3 out]
                        n596 = Format Into String(format string="%6.4f", w960) -> (resulting string=w961:string)  [unwired: 2 in, 1 out]
                        n597 = local write "Resulting string (W)"(w961) -> ()
                      }
                      frame #1 {
                        n598 = local read "Resulting string (W)"() -> (w969:string)
                        n599 = Concatenate Strings("Potencia_ajustada:", w969) -> (w967:string)
                        n600 = local write "Resulting string (W)"(w967) -> ()
                      }
                    }
                  }
                }
              }
              frame #5 {
                n601 = flat-sequence {
                  tunnel: [w983] -> w979
                  tunnel: [w981] -> w978
                  tunnel: w979 -> [w992]
                  tunnel: w978 -> [w991]
                  tunnel: [w990] -> w973
                  tunnel: [w989] -> w971
                  tunnel: w973 -> [w999]
                  tunnel: [w999] -> w972
                  tunnel: w971 -> [w998]
                  tunnel: [w998] -> w970
                  tunnel: w972 -> [w1003]
                  tunnel: w970 -> [w1002]
                  tunnel: [w1001] -> w977
                  tunnel: [w1000] -> w975
                  tunnel: w977 -> [w1010]
                  tunnel: [w1010] -> w976
                  tunnel: w975 -> [w1009]
                  tunnel: [w1009] -> w974
                  tunnel: w976 -> [w1014]
                  tunnel: w974 -> [w1013]
                  frame #0 {
                    n602 = Wait (ms)(milliseconds to wait=u32 10000) -> ()  [unwired: 1 out]
                  }
                  frame #1 {
                    w982 = u16 10 items=["1.0"=10, "1.5"=15, "2.0"=20] ("stop bits (10: 1 bit)")
                    (unwired) u8 13 ("termination char\n(0xA = '\\n' = LF)")
                    (unwired) u16 10 ("data bits (8)")
                    # "CONFIGURAÇÃO COMUNICAÇÃO PIC"
                    n603 = local read "COM PIC"() -> (w988:refnum<visa-resource-name>)
                    n604 = call-poly "VISA Configure Serial Port"("VISA resource name"=w988, "timeout (10sec)"=u32 120000, "Enable Termination\nChar (T)"=TRUE, "baud rate (9600)"=u32 9600, "parity (0:none)"=enum16{"None", "Odd", "Even", "Mark", "Space"}."None", "stop bits (10: 1 bit)"=w982) -> ("VISA resource name out"=w983:refnum<visa-resource-name>, "error out"=w981:errorcluster)  [unwired: 8 in]
                    n605 = local write "Erro comando PIC"(w981) -> ()
                  }
                  frame #2 {
                    # "FECHAMENTO OBTURADOR"
                    n606 = local write "Shutter ON (Verde)/ OFF (Vermelho)"(TRUE ("Inicia Controle")) -> ()
                    n607 = VISA Write(VISA resource name=w992, write buffer="F0000OK", error in (no error)=w991) -> (VISA resource name out=w990:refnum<visa-resource-name>, return count=w996:u32, error out=w989:errorcluster)
                    n608 = local write "return count"(w996) -> ()
                    n609 = local write "Motor Disco"(FALSE) -> ()
                    n610 = local write "Erro comando PIC"(w989) -> ()
                  }
                  frame #3 {
                    n611 = Wait (ms)(milliseconds to wait=u32 1000) -> ()  [unwired: 1 out]
                  }
                  frame #4 {
                    # "RETIRADA DO SENSOR"
                    n612 = local write "Shutter ON (Verde)/ OFF (Vermelho)"(TRUE) -> ()
                    n613 = VISA Write(VISA resource name=w1003, write buffer="R0000OK", error in (no error)=w1002) -> (VISA resource name out=w1001:refnum<visa-resource-name>, return count=w1004:u32, error out=w1000:errorcluster)
                    n614 = local write "return count"(w1004) -> ()
                    n615 = local write "Erro comando PIC"(w1000) -> ()
                    n616 = local write "Motor Sensor"(TRUE) -> ()
                  }
                  frame #5 {
                    n617 = Wait (ms)(milliseconds to wait=u32 5000) -> ()  [unwired: 1 out]
                  }
                  frame #6 {
                    # "ABERTURA DO OBTURADOR"
                    n618 = local write "Shutter ON (Verde)/ OFF (Vermelho)"(FALSE) -> ()
                    n619 = local write "Motor Sensor"(FALSE) -> ()
                    n620 = VISA Write(VISA resource name=w1014, write buffer="F0000OK", error in (no error)=w1013) -> (VISA resource name out=w1012:refnum<visa-resource-name>, return count=w1019:u32, error out=w1011:errorcluster)
                    n621 = local write "return count"(w1019) -> ()
                    n622 = property on="Setpoint (W)" class="DigNum (strict)"("DisabledEnum"=T2."Enabled" ("Disabled")) -> ()  [unwired: 2 in, 2 out]
                    n623 = VISA Close(VISA resource name=w1012, error in (no error)=w1011) -> ()  [unwired: 1 out]
                  }
                }
              }
              frame #6 {
                # "potencia_ajustada:0,0000(24caracteres)"
                # "AVISO AO USUÁRIO DE POTÊNCIA AJUSTADA"
                n624 = flat-sequence {
                  frame #0 {
                    n625 = local read "connection P3D ID out"() -> (w1022:refnum<k5>)
                    n626 = local read "Erro TCP 3DP"() -> (w1023:errorcluster)
                    n627 = while {
                      tunnel: [w1034] -> w1021
                      tunnel: [w1032] -> _
                      tunnel: w1022 -> [w1026]
                      tunnel: w1023 -> [w1025]
                      stop <- w1031 stop-if-true
                      n628 = local read "Resulting string (W)"() -> (w1027:string)
                      n629 = TCP Write(connection ID=w1026, data in=w1027, error in (no error)=w1025) -> (connection ID out=w1034:refnum<k5>, bytes written=w1030:i32, error out=w1032:errorcluster)  [unwired: 1 in]
                      n630 = Unbundle By Name(w1032) -> ("status"=w1033:bool)
                      n631 = Equal?(x=w1030, y=24) -> (x = y?=w1028:bool)
                      n632 = Or(x=w1033, y=w1028) -> (x .or. y?=w1031:bool)
                    }
                    n633 = local write "connection P3D ID out"(w1021) -> ()
                    n634 = Wait (ms)(milliseconds to wait=u32 500) -> ()  [unwired: 1 out]
                  }
                  frame #1 {
                    n635 = Wait (ms)(milliseconds to wait=u32 3000) -> ()  [unwired: 1 out]
                  }
                }
              }
            }
          }
          frame "Stop" {
            n636 = flat-sequence {
              frame #0 {
                n637 = local read "COM PIC"() -> (w1046:refnum<visa-resource-name>)
                n638 = call-poly "VISA Configure Serial Port"("VISA resource name"=w1046, "timeout (10sec)"=u32 10000, "termination char\n(0xA = '\\n' = LF)"=u8 10 ("termination char\n(0xA = '\\n' = LF)"), "Enable Termination\nChar (T)"=FALSE ("Enable Termination\nChar (T)"), "baud rate (9600)"=u32 9600, "data bits (8)"=u16 8, "parity (0:none)"=enum16{"None", "Odd", "Even", "Mark", "Space"}."None") -> ("VISA resource name out"=w1042:refnum<visa-resource-name>, "error out"=w1041:errorcluster)  [unwired: 7 in]
                n639 = VISA Write(VISA resource name=w1042, write buffer="F0000OK", error in (no error)=w1041) -> (VISA resource name out=w1040:refnum<visa-resource-name>, error out=w1039:errorcluster)  [unwired: 1 out]
                n640 = local write "Shutter ON (Verde)/ OFF (Vermelho)"(TRUE ("Inicia Controle")) -> ()
                n641 = VISA Write(VISA resource name=w1040, write buffer="S0000OK", error in (no error)=w1039) -> (VISA resource name out=w1044:refnum<visa-resource-name>, return count=w1043:u32, error out=w1045:errorcluster)
                n642 = local write "return count"(w1043) -> ()
                n643 = local write "Motor Sensor"(TRUE) -> ()
                n644 = VISA Close(VISA resource name=w1044, error in (no error)=w1045) -> ()  [unwired: 1 out]
              }
              frame #1 {
                n645 = local write "Mensagem de erro renviada"("Ops! Algo deu errado...") -> ()
              }
              frame #2 {
                n646 = local read "connection P3D ID out"() -> (w1058:refnum<k5>)
                n647 = local read "Erro TCP 3DP"() -> (w1059:errorcluster)
                n648 = TCP Write(connection ID=w1058, data in="Mensagem de erro renviada", error in (no error)=w1059) -> ()  [unwired: 1 in, 3 out]
              }
            }
            n649 = property on="Setpoint (W)" class="DigNum (strict)"("DisabledEnum"=T2."Disabled" ("Disabled")) -> ()  [unwired: 2 in, 2 out]
          }
        }
      }
      event "Quit": Value Change {
        w1060 = "Encerra Programa?" ("message")
        n650 = event-data() -> ()  [unwired: 1 in, 5 out]
        n651 = local write "Mensagem de erro renviada"(w1060) -> ()
        n652 = Two Button Dialog(message=w1060, 1:"Não" ("F button name (\"Cancel\")"), 2:"Sim" ("T button name (\"OK\")")) -> (T button?=w1066:bool)
        n653 = Select(t=TCC_01_02_15."Stop", s=w1066, f=TCC_01_02_15."Receber Potencia") -> (s? t:f=w1061:T1)
      }
      event "Erro comando PIC": Value Change {
        n654 = event-data() -> ()  [unwired: 1 in, 5 out]
      }
      event "Inicia Controle": Value Change {
        n655 = event-data() -> ()  [unwired: 1 in, 5 out]
        n656 = Two Button Dialog(message="Braçal mesmo?", 1:"Melhor esperar o orientador..." ("F button name (\"Cancel\")"), 2:"Certeza!" ("T button name (\"OK\")")) -> (T button?=w1071:bool)
        n657 = Select(t=TCC_01_02_15."Limites_Manual" ("States"), s=w1071, f=TCC_01_02_15."Eventos" ("States")) -> (s? t:f=w1068:T1)
      }
    }
    n658 = Equal?(x=w5, y=TCC_01_02_15."Stop" ("States")) -> (x = y?=w7:bool)
    n659 = Wait (ms)(milliseconds to wait=u32 125) -> ()  [unwired: 1 out]
  }
